vi "Configure.vi"(8 "error in (no error)":errorcluster, 10 "Msg in":T2, 11 "FakePressureController in":refnum<class "Tapedrive_ESP301.lvclass">) -> (0 "error out":errorcluster, 1 "new command":string, 2 "Msg out":T2, 3 "FakePressureController out":refnum<class "Tapedrive_ESP301.lvclass">)   [LabVIEW 2013, in "Tapedrive_ESP301.lvclass"]
uses:
  Tapedrive_ESP301.lvclass
  shared/OnOffTypeDef.ctl
  shared/CompressAndUpdate(Poly)/CompressAndUpdate(Numeric).vi
  shared/CompressAndUpdate(Poly)/CompressAndUpdate(Enum).vi
  shared/CompressAndUpdate(Poly)/CompressAndUpdate(String).vi
  BaseDriver/BaseDriver.lvclass
  BaseDriver/DriverMsg.ctl
panel:
  out "Error Code":i32[](array[numeric])
  out "Error Message":string
  out "velo":dbl(graph)
  out "Position (units)":dbl(graph)
  out "spreadsheet string":string
  out "found?":bool
  out "Settings.Velocity":T1
  out "Channel":string
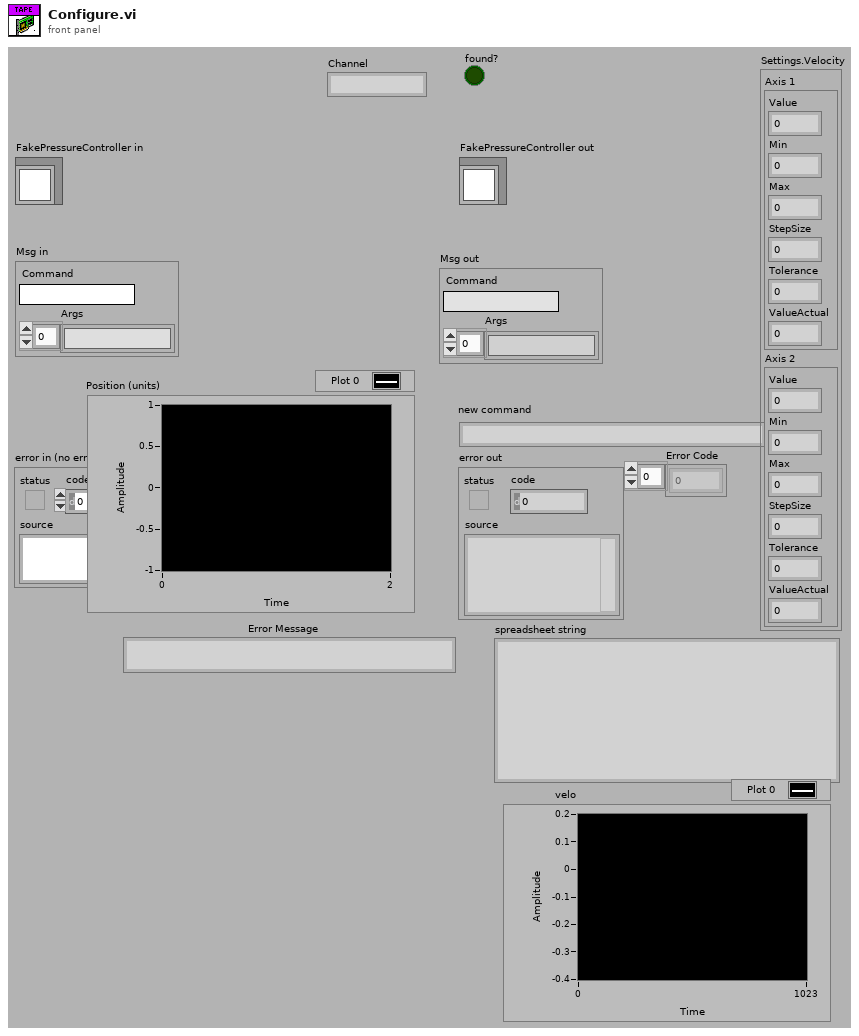
[diagram p1: front panel]
types:
  T1 = cluster{"Axis 1":cluster{"Value":dbl, "Min":dbl, "Max":dbl, "StepSize":dbl, "Tolerance":dbl, "ValueActual":dbl}, "Axis 2":cluster{"Value":dbl, "Min":dbl, "Max":dbl, "StepSize":dbl, "Tolerance":dbl, "ValueActual":dbl}}
  T2 = typedef "DriverMsg.ctl" = cluster{"Command":string, "Args":string[]}
  T3 = typedef "OnOffTypeDef.ctl" = enum16{"off", "on"}
  T4 = enum16{"Not referenced", "Homing", "Moving", "Ready"}
  T5 = typedef "Direction.ctl" = enum16{"Forward", "Backward", "Undefined"}
  T6 = typedef "Tapedrive_ESP301.lvclass/settingsCluster_TapeDrive_TypDef.ctl" = cluster{"devport":string, "tapepos":cluster{"Value":dbl, "Min":dbl, "Max":dbl, "StepSize":dbl, "Tolerance":dbl, "ValueActual":dbl}, "status":enum16{"Not referenced", "Homing", "Moving", "Ready"}, "inmotion":T3, "forwardaxis":i16, "backwardaxis":i16, "encoderaxis":i16, "Velocity":cluster{"Axis 1":cluster{"Value":dbl, "Min":dbl, "Max":dbl, "StepSize":dbl, "Tolerance":dbl, "ValueActual":dbl}, "Axis 2":cluster{"Value":dbl, "Min":dbl, "Max":dbl, "StepSize":dbl, "Tolerance":dbl, "ValueActual":dbl}}, "Acceleration":cluster{"Axis 1":cluster{"Value":dbl, "Min":dbl, "Max":dbl, "StepSize":dbl, "Tolerance":dbl, "ValueActual":dbl}, "Axis 2":cluster{"Value":dbl, "Min":dbl, "Max":dbl, "StepSize":dbl, "Tolerance":dbl, "ValueActual":dbl}}, "Decceleration":cluster{"Axis 1":cluster{"Value":dbl, "Min":dbl, "Max":dbl, "StepSize":dbl, "Tolerance":dbl, "ValueActual":dbl}, "Axis 2":cluster{"Value":dbl, "Min":dbl, "Max":dbl, "StepSize":dbl, "Tolerance":dbl, "ValueActual":dbl}}, "MaxAcceleration":cluster{"Axis 1":cluster{"Value":dbl, "Min":dbl, "Max":dbl, "StepSize":dbl, "Tolerance":dbl, "ValueActual":dbl}, "Axis 2":cluster{"Value":dbl, "Min":dbl, "Max":dbl, "StepSize":dbl, "Tolerance":dbl, "ValueActual":dbl}}, "MaxVelocity":cluster{"Axis 1":cluster{"Value":dbl, "Min":dbl, "Max":dbl, "StepSize":dbl, "Tolerance":dbl, "ValueActual":dbl}, "Axis 2":cluster{"Value":dbl, "Min":dbl, "Max":dbl, "StepSize":dbl, "Tolerance":dbl, "ValueActual":dbl}}, "VelocityFFG":cluster{"Axis 1":cluster{"Value":dbl, "Min":dbl, "Max":dbl, "StepSize":dbl, "Tolerance":dbl, "ValueActual":dbl}, "Axis 2":cluster{"Value":dbl, "Min":dbl, "Max":dbl, "StepSize":dbl, "Tolerance":dbl, "ValueActual":dbl}}, "AccelerationFFG":cluster{"Axis 1":cluster{"Value":dbl, "Min":dbl, "Max":dbl, "StepSize":dbl, "Tolerance":dbl, "ValueActual":dbl}, "Axis 2":cluster{"Value":dbl, "Min":dbl, "Max":dbl, "StepSize":dbl, "Tolerance":dbl, "ValueActual":dbl}}, "DACoffset":cluster{"Axis 1":cluster{"Value":dbl, "Min":dbl, "Max":dbl, "StepSize":dbl, "Tolerance":dbl, "ValueActual":dbl}, "Axis 2":cluster{"Value":dbl, "Min":dbl, "Max":dbl, "StepSize":dbl, "Tolerance":dbl, "ValueActual":dbl}}, "Power":cluster{"Axis 1":T3, "Axis 2":T3}, "ReductionRatio":cluster{"Value":dbl, "Min":dbl, "Max":dbl, "StepSize":dbl, "Tolerance":dbl, "ValueActual":dbl}, "Direction":T5, "Tension":T3, "TensionVelocity":cluster{"Axis 1":cluster{"Value":dbl, "Min":dbl, "Max":dbl, "StepSize":dbl, "Tolerance":dbl, "ValueActual":dbl}, "Axis 2":cluster{"Value":dbl, "Min":dbl, "Max":dbl, "StepSize":dbl, "Tolerance":dbl, "ValueActual":dbl}}, "TensionAcceleration":cluster{"Axis 1":cluster{"Value":dbl, "Min":dbl, "Max":dbl, "StepSize":dbl, "Tolerance":dbl, "ValueActual":dbl}, "Axis 2":cluster{"Value":dbl, "Min":dbl, "Max":dbl, "StepSize":dbl, "Tolerance":dbl, "ValueActual":dbl}}, "TensionDecceleration":cluster{"Axis 1":cluster{"Value":dbl, "Min":dbl, "Max":dbl, "StepSize":dbl, "Tolerance":dbl, "ValueActual":dbl}, "Axis 2":cluster{"Value":dbl, "Min":dbl, "Max":dbl, "StepSize":dbl, "Tolerance":dbl, "ValueActual":dbl}}, "MoveVelocity":cluster{"Axis 1":cluster{"Value":dbl, "Min":dbl, "Max":dbl, "StepSize":dbl, "Tolerance":dbl, "ValueActual":dbl}, "Axis 2":cluster{"Value":dbl, "Min":dbl, "Max":dbl, "StepSize":dbl, "Tolerance":dbl, "ValueActual":dbl}}, "MoveAcceleration":cluster{"Axis 1":cluster{"Value":dbl, "Min":dbl, "Max":dbl, "StepSize":dbl, "Tolerance":dbl, "ValueActual":dbl}, "Axis 2":cluster{"Value":dbl, "Min":dbl, "Max":dbl, "StepSize":dbl, "Tolerance":dbl, "ValueActual":dbl}}, "MoveDecceleration":cluster{"Axis 1":cluster{"Value":dbl, "Min":dbl, "Max":dbl, "StepSize":dbl, "Tolerance":dbl, "ValueActual":dbl}, "Axis 2":cluster{"Value":dbl, "Min":dbl, "Max":dbl, "StepSize":dbl, "Tolerance":dbl, "ValueActual":dbl}}, "MaxStepsize":cluster{"Value":dbl, "Min":dbl, "Max":dbl, "StepSize":dbl, "Tolerance":dbl, "ValueActual":dbl}, "Stepsize":cluster{"Value":dbl, "Min":dbl, "Max":dbl, "StepSize":dbl, "Tolerance":dbl, "ValueActual":dbl}, "GoStep":T3, "StopWait":T3, "stepnum":cluster{"Value":dbl, "Min":dbl, "Max":dbl, "StepSize":dbl, "Tolerance":dbl, "ValueActual":dbl}, "MoveIfScan":T3, "HomeEncoder":T3, "Timeout":cluster{"Value":dbl, "Min":dbl, "Max":dbl, "StepSize":dbl, "Tolerance":dbl, "ValueActual":dbl}, "TapeRelax":cluster{"Value":dbl, "Min":dbl, "Max":dbl, "StepSize":dbl, "Tolerance":dbl, "ValueActual":dbl}}
  T7 = cluster{"Axis 1":cluster{"Value":dbl, "Min":dbl, "Max":dbl, "StepSize":dbl, "Tolerance":dbl, "ValueActual":dbl}, "Axis 2":cluster{"Value":dbl, "Min":dbl, "Max":dbl, "StepSize":dbl, "Tolerance":dbl, "ValueActual":dbl}}[]
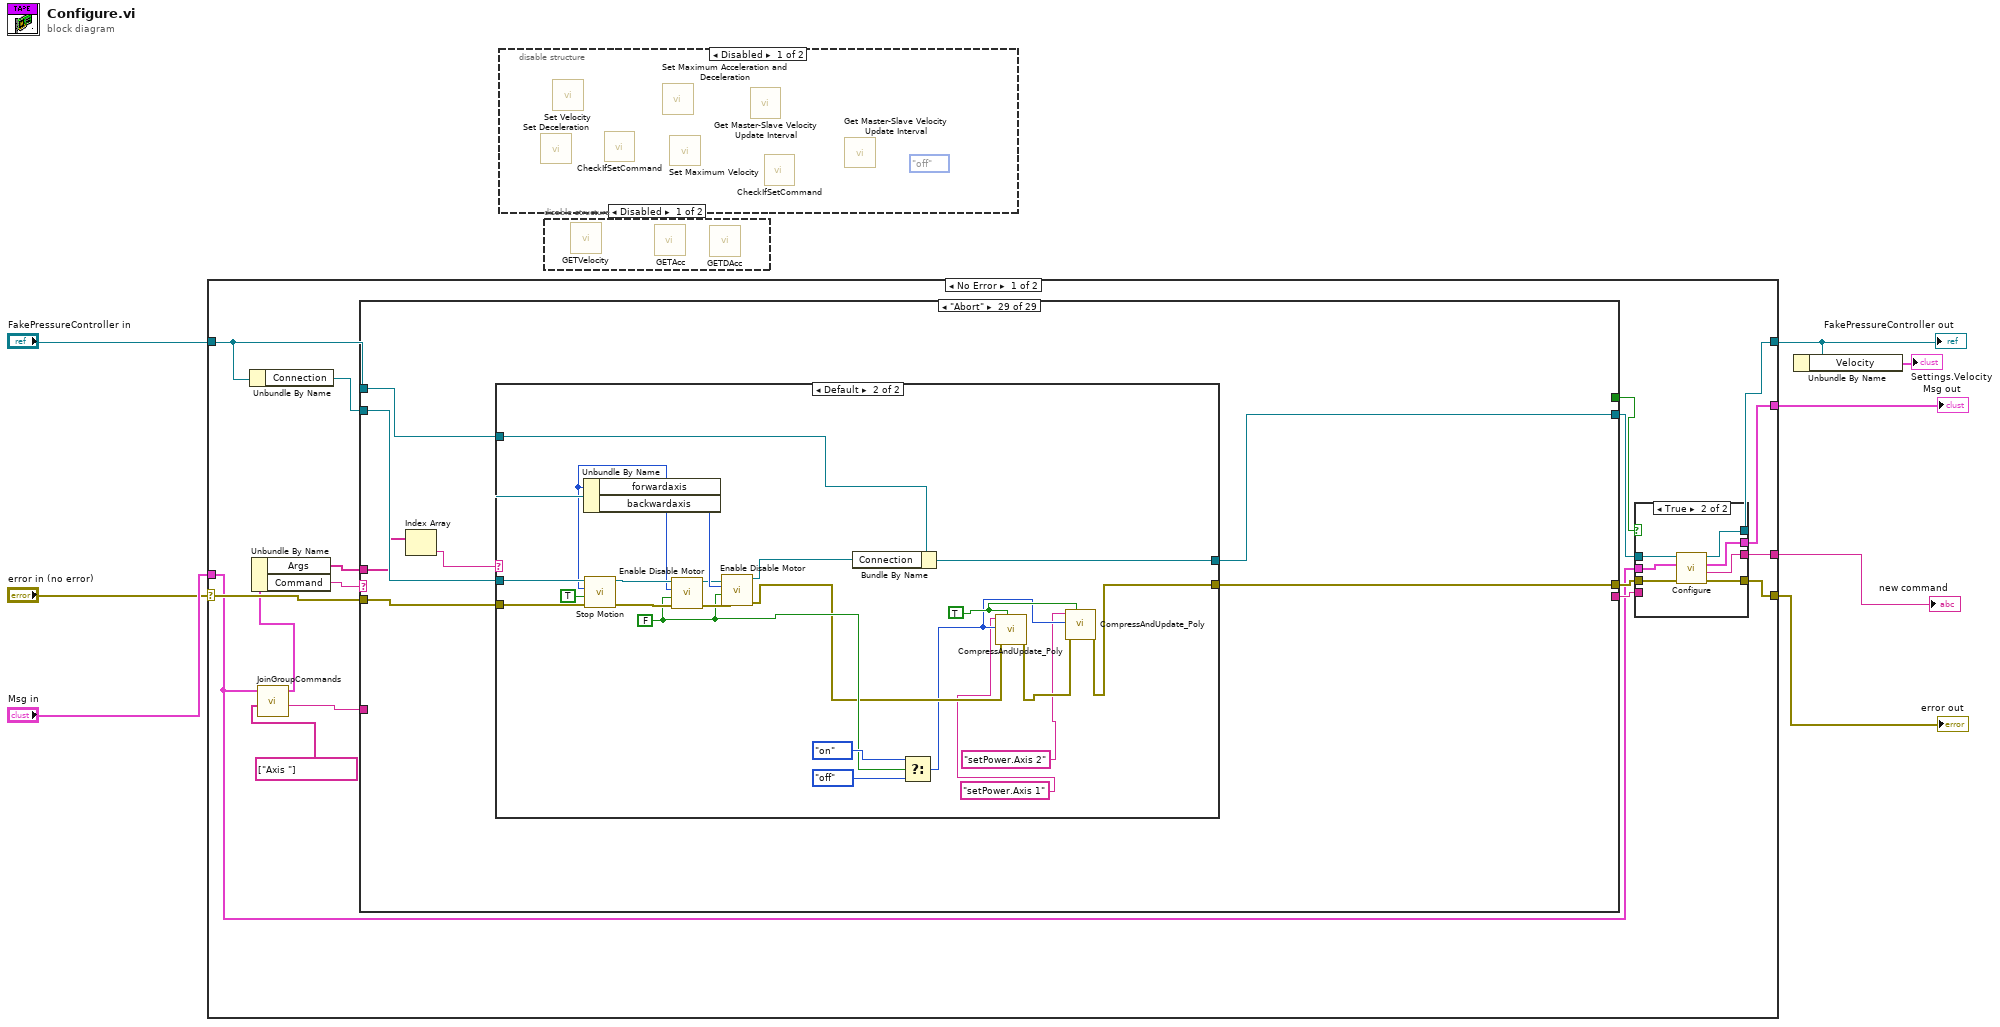
[diagram p0: block diagram]
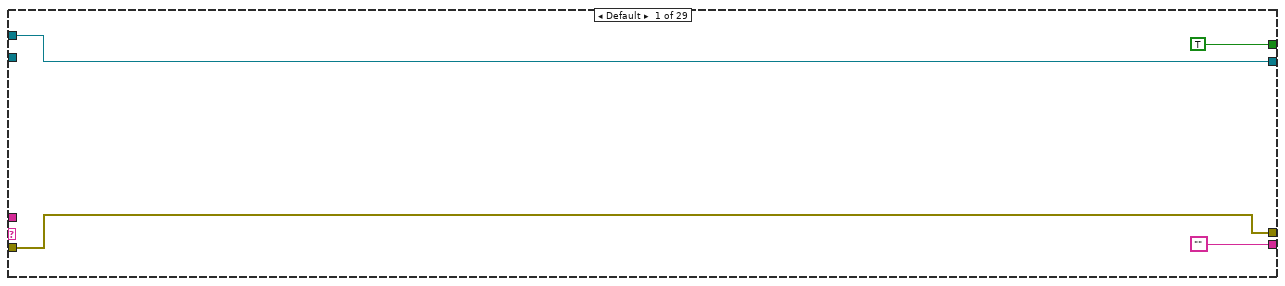
[diagram p5: hidden frame]
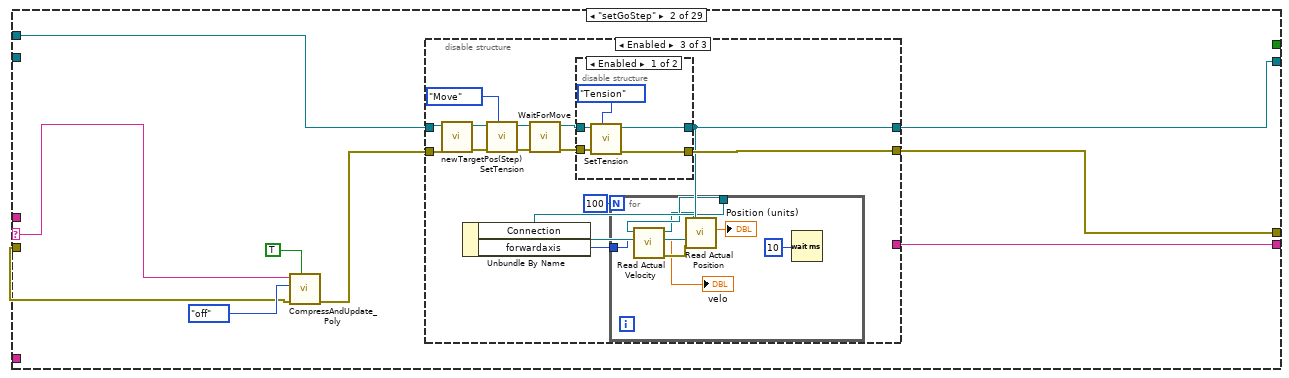
[diagram p6: hidden frame]
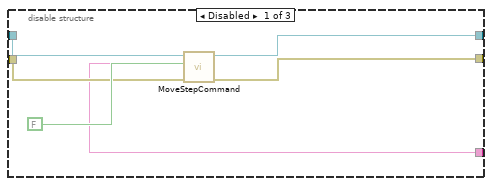
[diagram p7: hidden frame]
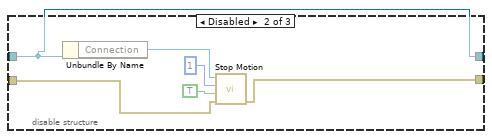
[diagram p8: hidden frame]
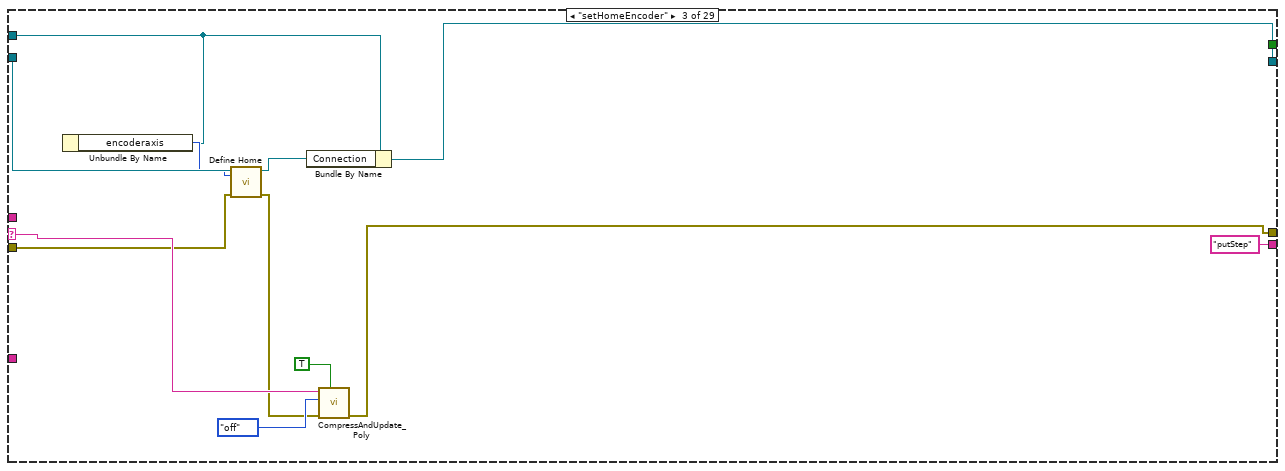
[diagram p10: hidden frame]
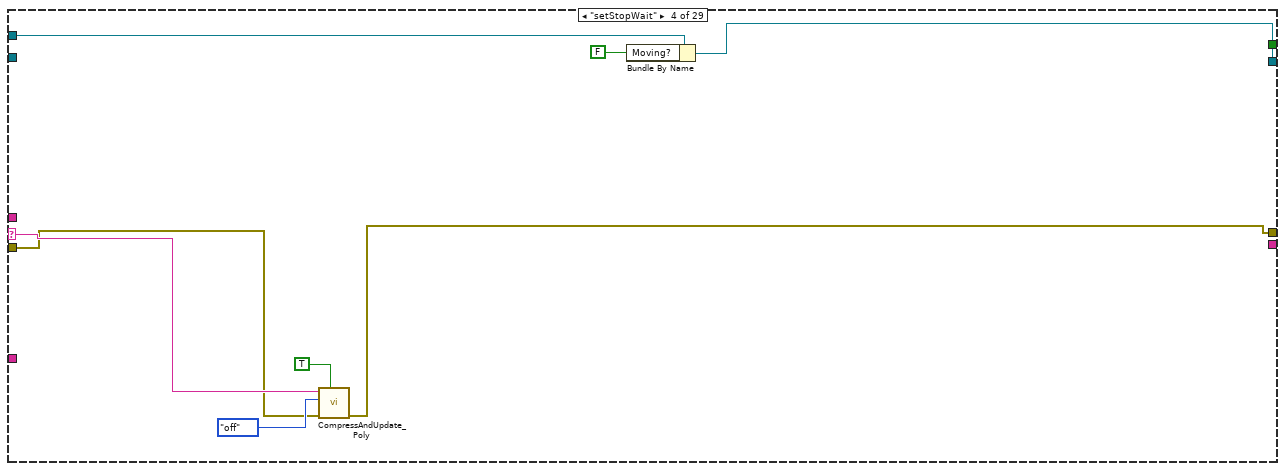
[diagram p11: hidden frame]
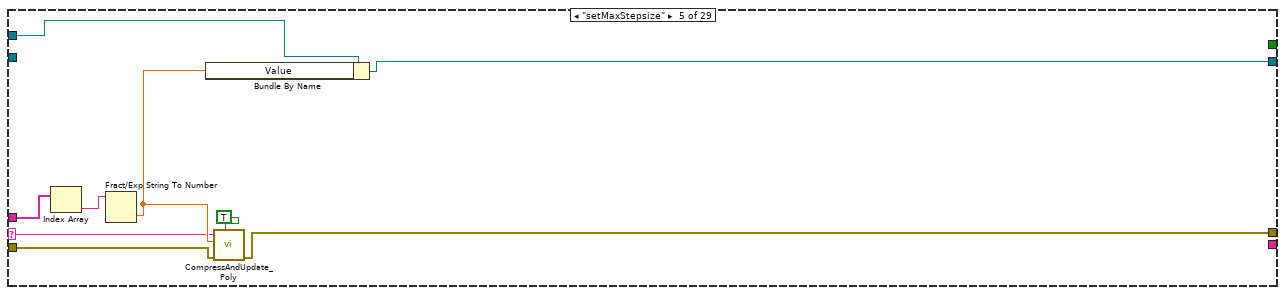
[diagram p12: hidden frame]
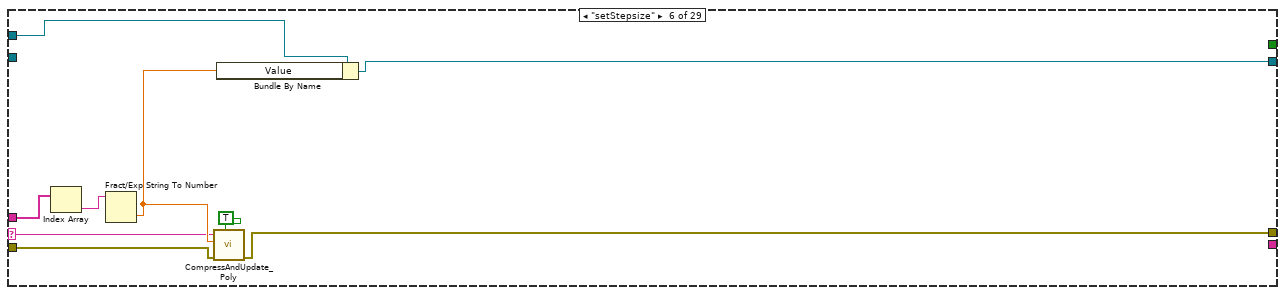
[diagram p13: hidden frame]
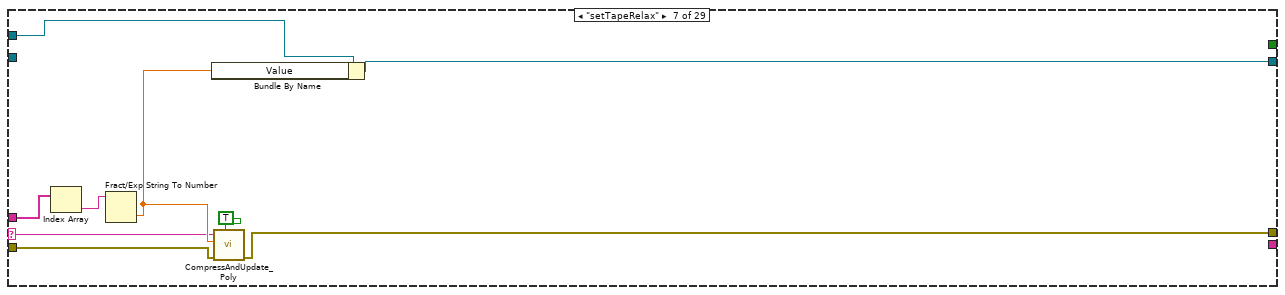
[diagram p14: hidden frame]
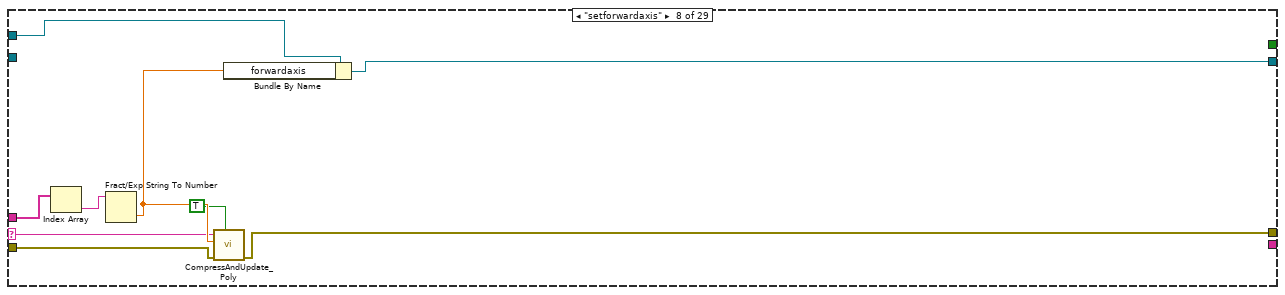
[diagram p15: hidden frame]
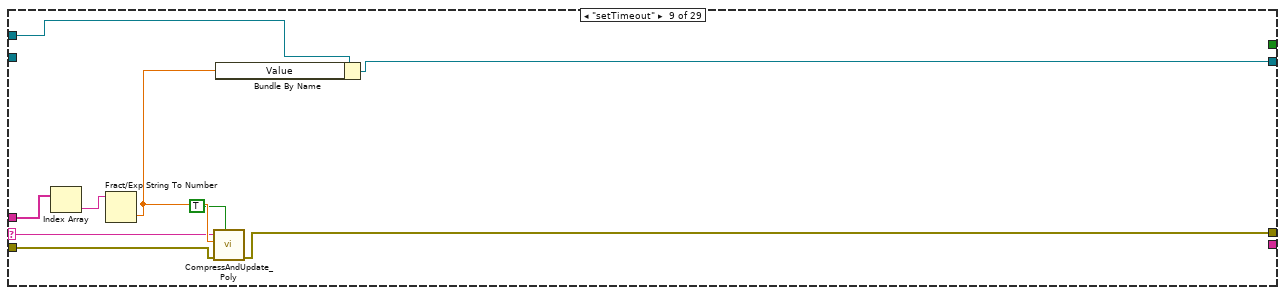
[diagram p16: hidden frame]
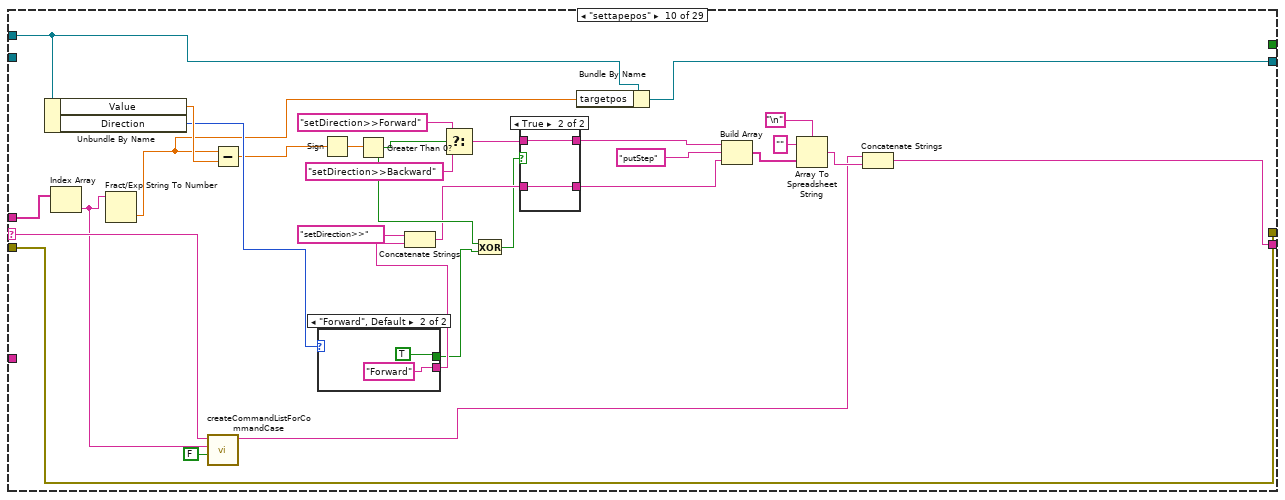
[diagram p17: hidden frame]
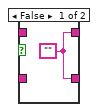
[diagram p18: hidden frame]
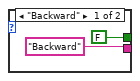
[diagram p19: hidden frame]
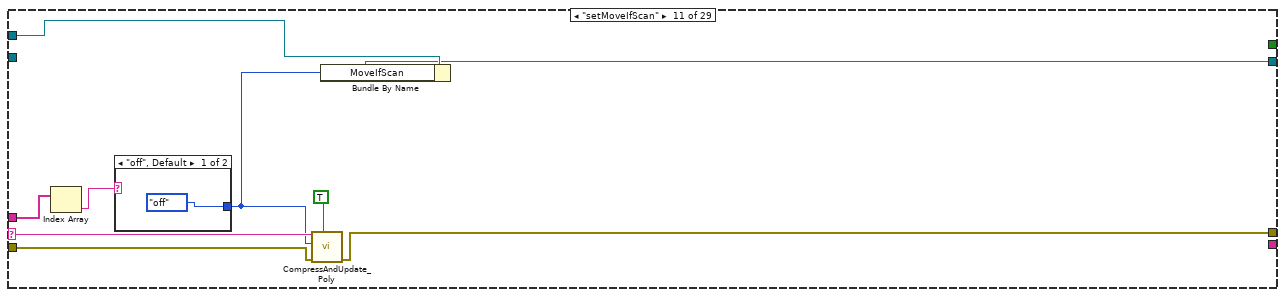
[diagram p20: hidden frame]
diagram:
  n1 = case shown="No Error" "error in (no error)" {
    selector: "error in (no error)" -> [w17 w958]
    tunnel: "FakePressureController in" -> [w14 w956]
    tunnel: [w24 w956] -> w2
    tunnel: [w22 w958] -> w5
    tunnel: "Msg in" -> [w9 w957]
    tunnel: [w20 w957] -> w4
    tunnel: [w18 _] -> w3
    frame No Error {
      n2 = Unbundle By Name(w14) -> ("Connection"=w13:refnum<visa-resource-name>)
      n3 = call "JoinGroupCommands.vi"("Seperator"=string[] ["Axis "], "Msg in"=w9) -> ("Seperator out"=w10:string, "Msg out"=w12:T2)  [unwired: 7 in, 1 out]
      n4 = Unbundle By Name(w12) -> ("Args"=w16:string[], "Command"=w15:string)
      n5 = case shown="\"Abort\"" w15 {
        selector: w15 -> [_ w42 w99 w108 w112 w121 w130 w139 w148 w172 w196 w205 w214 w224 w238 w270 w456 w480 w504 w687 w717 _ _ _ _ w803 _ _ _]
        tunnel: w17 -> [w39 w47 w93 w105 w111 w120 w129 w138 w147 w182 w195 w204 w213 w223 w229 w278 w465 w476 w506 w676 w701 w721 w727 w732 w742 w815 w830 w902 w928]
        tunnel: w16 -> [_ _ _ _ w115 w124 w133 w142 w151 w183 w197 w208 w217 w225 w240 w277 w464 w487 w515 w673 w708 w723 _ w731 _ w814 _ w905 w926]
        tunnel: w14 -> [w40 w45 w91 w103 w117 w126 w135 w144 w153 w177 w199 w210 w219 w227 w232 w260 w458 w483 w493 w680 w693 w720 w726 w733 w737 w811 w825 w897 w930]
        tunnel: [w40 w44 w90 w102 w116 w125 w134 w143 w152 w176 w198 w209 w218 w226 w241 w271 w457 w481 w508 w678 w709 w719 w725 w733 w734 w810 w822 w888 w931] -> w25
        tunnel: ["" ("Complete") w41 "putStep" ("spreadsheet string") _ _ _ _ _ _ w167 _ _ _ _ w235 w264 w440 w477 w509 w681 w711 _ _ _ w743 _ w831 w900 _] -> w19
        tunnel: [w39 w46 w96 w104 w110 w119 w128 w137 w146 w182 w194 w203 w212 w222 w234 w259 w443 w475 w491 w662 w698 w718 w724 w732 w736 w804 w824 w889 w927] -> w23
        tunnel: [TRUE _ _ _ _ _ _ _ _ _ _ _ _ _ _ _ _ _ _ _ _ _ _ _ _ _ _ _ _] -> w21
        tunnel: w13 -> [_ _ w95 _ _ _ _ _ _ _ _ _ _ _ w231 w279 w466 _ w505 w677 w702 _ _ _ w740 w819 w828 w904 w929]
        tunnel: w10 -> [_ _ _ _ _ _ _ _ _ _ _ _ _ _ _ w275 w462 _ w513 w685 w715 _ _ _ _ _ _ _ _]
        frame Default {
        }
        frame "setGoStep" {
          n6 = call-poly "CompressAndUpdate_Poly.vi"("force CVT update (false)"=TRUE, "error in"=w47, "enum variant"=OnOffTypeDef."off" ("inmotion"), "command or variable name"=w42) -> ("error out"=w43:errorcluster)  [unwired: 7 in]
          n7 = disable-structure shown="Enabled" {
            disable-tunnel: [w55 w56 w72] -> w46
            disable-tunnel: w45 -> [w54 w59 w67]
            disable-tunnel: [w53 w59 w64] -> w44
            disable-tunnel: w43 -> [w51 w57 w74]
            disable-tunnel: [w50 _ _] -> w41
            frame Disabled {
              n8 = call "MoveStepCommand.vi"("error in (no error)"=w51, "MultiCVT"=FALSE, "Tapedrive_ESP301 in"=w54) -> ("error out"=w55:errorcluster, "String"=w50:string, "Tapedrive_ESP301.lvclass"=w53:refnum<class "Tapedrive_ESP301.lvclass">)  [unwired: 6 in]
            }
            frame Disabled {
              n9 = Unbundle By Name(w59) -> ("Connection"=w58:refnum<visa-resource-name>)
              n10 = call <instrlib>:"Stop Motion.vi"("error in (no error)"=w57, "Stop all axes (F)"=TRUE, "Axis (1)"=1, "VISA resource name"=w58) -> ("error out"=w56:errorcluster)  [unwired: 2 in, 1 out]
            }
            frame Enabled {
              n11 = call "newTargetPos(Step).vi"("Tapedrive_ESP301 in"=w67) -> ("Tapedrive_ESP301 out"=w66:refnum<class "Tapedrive_ESP301.lvclass">)  [unwired: 9 in, 1 out]
              n12 = call "SetTension.vi"("command"=enum16{"Move", "Tension"}."Move", "error in (no error)"=w74, "Tapedrive_ESP301 in"=w66) -> ("error out"=w69:errorcluster, "Tapedrive_ESP301 out"=w71:refnum<class "Tapedrive_ESP301.lvclass">)  [unwired: 7 in]
              n13 = call-dynamic "WaitForMove.vi"("error in (no error)"=w69, "Tapedrive Object"=w71) -> ("error out (no error)"=w68:errorcluster, "Tapedrive Object 2"=w70:refnum<class "Tapedrive_ESP301.lvclass">)  [unwired: 7 in, 1 out]
              n14 = disable-structure shown="Enabled" {
                disable-tunnel: [w86 w88] -> w64
                disable-tunnel: [w84 w87] -> w72
                disable-tunnel: w70 -> [w83 w88]
                disable-tunnel: w68 -> [w82 w87]
                frame Enabled {
                  n15 = call "SetTension.vi"("command"=enum16{"Move", "Tension"}."Tension", "error in (no error)"=w82, "Tapedrive_ESP301 in"=w83) -> ("error out"=w84:errorcluster, "Tapedrive_ESP301 out"=w86:refnum<class "Tapedrive_ESP301.lvclass">)  [unwired: 7 in]
                }
                frame Disabled {
                }
              }
              n16 = Unbundle By Name(w64) -> ("Connection"=w63:refnum<visa-resource-name>, "forwardaxis"=w62:i16)
              n17 = for {
                N: 100 -> [_]
                tunnel: w63 -> [w78]
                tunnel: w62 -> [w76]
                n18 = call <instrlib>:"Read Actual Velocity.vi"("Axis (1)"=w76, "VISA resource name"=w78) -> ("error out"=w79:errorcluster, "Velocity (units/s)"=→"velo":dbl, "VISA resource name out"=w77:refnum<visa-resource-name>)  [unwired: 3 in]
                n19 = call <instrlib>:"Read Actual Position.vi"("error in (no error)"=w79, "VISA resource name"=w77) -> ("Position (units)"=→"Position (units)":dbl)  [unwired: 3 in, 2 out]
                n20 = Wait (ms)(milliseconds to wait=u32 10) -> ()  [unwired: 1 out]
              }
            }
          }
        }
        frame "setHomeEncoder" {
          n21 = Unbundle By Name(w91) -> ("encoderaxis"=w94:i16)
          n22 = call <instrlib>:"Define Home.vi"("error in (no error)"=w93, "Axis (1)"=w94, "VISA resource name"=w95) -> ("error out"=w92:errorcluster, "VISA resource name out"=w89:refnum<visa-resource-name>)  [unwired: 3 in]
          n23 = Bundle By Name(cluster=w91, "Connection"=w89) -> (w90:refnum<class "Tapedrive_ESP301.lvclass">)
          n24 = call-poly "CompressAndUpdate_Poly.vi"("force CVT update (false)"=TRUE, "error in"=w92, "enum variant"=OnOffTypeDef."off" ("inmotion"), "command or variable name"=w99) -> ("error out"=w96:errorcluster)  [unwired: 7 in]
        }
        frame "setStopWait" {
          n25 = call-poly "CompressAndUpdate_Poly.vi"("force CVT update (false)"=TRUE, "error in"=w105, "enum variant"=OnOffTypeDef."off" ("inmotion"), "command or variable name"=w108) -> ("error out"=w104:errorcluster)  [unwired: 7 in]
          n26 = Bundle By Name(cluster=w103, "Moving?"=FALSE ("Wait for Step")) -> (w102:refnum<class "Tapedrive_ESP301.lvclass">)
        }
        frame "setMaxStepsize" {
          n27 = Index Array(array=w115) -> (element=w114:string)  [unwired: 1 in]
          n28 = Fract/Exp String To Number(string=w114) -> (number=w113:dbl)  [unwired: 3 in, 1 out]
          n29 = Bundle By Name(cluster=w117, "Value"=w113) -> (w116:refnum<class "Tapedrive_ESP301.lvclass">)
          n30 = call-poly "CompressAndUpdate_Poly.vi"("force CVT update (false)"=TRUE, "error in"=w111, "Numeric"=w113, "command or variable name"=w112) -> ("error out"=w110:errorcluster)  [unwired: 7 in]
        }
        frame "setStepsize" {
          n31 = Index Array(array=w124) -> (element=w123:string)  [unwired: 1 in]
          n32 = Fract/Exp String To Number(string=w123) -> (number=w122:dbl)  [unwired: 3 in, 1 out]
          n33 = call-poly "CompressAndUpdate_Poly.vi"("force CVT update (false)"=TRUE, "error in"=w120, "Numeric"=w122, "command or variable name"=w121) -> ("error out"=w119:errorcluster)  [unwired: 7 in]
          n34 = Bundle By Name(cluster=w126, "Value"=w122) -> (w125:refnum<class "Tapedrive_ESP301.lvclass">)
        }
        frame "setTapeRelax" {
          n35 = Index Array(array=w133) -> (element=w132:string)  [unwired: 1 in]
          n36 = Fract/Exp String To Number(string=w132) -> (number=w131:dbl)  [unwired: 3 in, 1 out]
          n37 = Bundle By Name(cluster=w135, "Value"=w131) -> (w134:refnum<class "Tapedrive_ESP301.lvclass">)
          n38 = call-poly "CompressAndUpdate_Poly.vi"("force CVT update (false)"=TRUE, "error in"=w129, "Numeric"=w131, "command or variable name"=w130) -> ("error out"=w128:errorcluster)  [unwired: 7 in]
        }
        frame "setforwardaxis" {
          n39 = Index Array(array=w142) -> (element=w141:string)  [unwired: 1 in]
          n40 = Fract/Exp String To Number(string=w141) -> (number=w140:dbl)  [unwired: 3 in, 1 out]
          n41 = call-poly "CompressAndUpdate_Poly.vi"("force CVT update (false)"=TRUE, "error in"=w138, "Numeric"=w140, "command or variable name"=w139) -> ("error out"=w137:errorcluster)  [unwired: 7 in]
          n42 = Bundle By Name(cluster=w144, "forwardaxis"=w140) -> (w143:refnum<class "Tapedrive_ESP301.lvclass">)
        }
        frame "setTimeout" {
          n43 = Index Array(array=w151) -> (element=w150:string)  [unwired: 1 in]
          n44 = Fract/Exp String To Number(string=w150) -> (number=w149:dbl)  [unwired: 3 in, 1 out]
          n45 = call-poly "CompressAndUpdate_Poly.vi"("force CVT update (false)"=TRUE, "error in"=w147, "Numeric"=w149, "command or variable name"=w148) -> ("error out"=w146:errorcluster)  [unwired: 7 in]
          n46 = Bundle By Name(cluster=w153, "Value"=w149) -> (w152:refnum<class "Tapedrive_ESP301.lvclass">)
        }
        frame "settapepos" {
          n47 = Unbundle By Name(w177) -> ("Value"=w181:dbl, "Direction"=w164:T5)
          n48 = Index Array(array=w183) -> (element=w171:string)  [unwired: 1 in]
          n49 = Fract/Exp String To Number(string=w171) -> (number=w155:dbl)  [unwired: 3 in, 1 out]
          n50 = call "createCommandListForCommandCase.vi"("immediate Check (only once)"=FALSE, "setvalue"=w171, "command"=w172) -> ("new commands"=w168:string)  [unwired: 8 in]
          n51 = Subtract(x=w155, y=w181) -> (x-y=w154:dbl)
          n52 = case shown="\"Forward\", Default" w164 {
            tunnel: ["Backward" "Forward"] -> w163
            tunnel: [FALSE TRUE] -> w161
            frame "Backward" {
            }
            frame "Forward", Default {
            }
          }
          n53 = Sign(1:w154) -> (0:w180:dbl)
          n54 = Greater Than 0?(x=w180) -> (x > 0?=w162:bool)
          n55 = Concatenate Strings("setDirection>>", w163) -> (w158:string)
          n56 = Select(t="setDirection>>Forward", s=w162, f="setDirection>>Backward") -> (s? t:f=w160:string)
          n57 = Exclusive Or(1:w161, 2:w162) -> (0:w156:bool)
          n58 = case shown="True" w156 {
            tunnel: w160 -> [_ w186]
            tunnel: [w184 w186] -> w159
            tunnel: w158 -> [_ w185]
            tunnel: [w184 w185] -> w157
            frame False {
              w184 = ""
            }
            frame True {
            }
          }
          n59 = Bundle By Name(cluster=w177, "targetpos"=w155) -> (w176:refnum<class "Tapedrive_ESP301.lvclass">)
          n60 = Build Array(w159, "putStep", w157) -> (w175:string[])
          n61 = Array To Spreadsheet String(delimiter (Tab)="\n", array=w175, 3:"" ("format string")) -> (spreadsheet string=w169:string)
          n62 = Concatenate Strings(w168, w169) -> (w167:string)
        }
        frame "setMoveIfScan" {
          n63 = Index Array(array=w197) -> (element=w192:string)  [unwired: 1 in]
          n64 = case shown="\"off\", Default" w192 {
            tunnel: [OnOffTypeDef."off" ("inmotion") OnOffTypeDef."on" ("inmotion")] -> w191
            frame "off", Default {
            }
            frame "on" {
            }
          }
          n65 = call-poly "CompressAndUpdate_Poly.vi"("force CVT update (false)"=TRUE, "error in"=w195, "enum variant"=w191, "command or variable name"=w196) -> ("error out"=w194:errorcluster)  [unwired: 7 in]
          n66 = Bundle By Name(cluster=w199, "MoveIfScan"=w191) -> (w198:refnum<class "Tapedrive_ESP301.lvclass">)
        }
        frame "setbackwardaxis" {
          n67 = Index Array(array=w208) -> (element=w207:string)  [unwired: 1 in]
          n68 = Fract/Exp String To Number(string=w207) -> (number=w206:dbl)  [unwired: 3 in, 1 out]
          n69 = call-poly "CompressAndUpdate_Poly.vi"("force CVT update (false)"=TRUE, "error in"=w204, "Numeric"=w206, "command or variable name"=w205) -> ("error out"=w203:errorcluster)  [unwired: 7 in]
          n70 = Bundle By Name(cluster=w210, "backwardaxis"=w206) -> (w209:refnum<class "Tapedrive_ESP301.lvclass">)
        }
        frame "setencoderaxis" {
          n71 = Index Array(array=w217) -> (element=w216:string)  [unwired: 1 in]
          n72 = Fract/Exp String To Number(string=w216) -> (number=w215:dbl)  [unwired: 3 in, 1 out]
          n73 = call-poly "CompressAndUpdate_Poly.vi"("force CVT update (false)"=TRUE, "error in"=w213, "Numeric"=w215, "command or variable name"=w214) -> ("error out"=w212:errorcluster)  [unwired: 7 in]
          n74 = Bundle By Name(cluster=w219, "encoderaxis"=w215) -> (w218:refnum<class "Tapedrive_ESP301.lvclass">)
        }
        frame "setdevport" {
          n75 = Index Array(array=w225) -> (element=w221:string)  [unwired: 1 in]
          n76 = call-poly "CompressAndUpdate_Poly.vi"("force CVT update (false)"=TRUE, "error in"=w223, "String"=w221, "command or variable name"=w224) -> ("error out"=w222:errorcluster)  [unwired: 7 in]
          n77 = Bundle By Name(cluster=w227, "devport"=w221) -> (w226:refnum<class "Tapedrive_ESP301.lvclass">)
        }
        frame "setTension" {
          # "TODO: tension off??"
          n78 = Index Array(array=w240) -> (element=w237:string)  [unwired: 1 in]
          n79 = Unbundle By Name(w232) -> ("forwardaxis"=w230:i16)
          n80 = call "createCommandListForCommandCase.vi"("setvalue"=w237, "command"=w238) -> ("new commands"=w236:string)  [unwired: 9 in]
          n81 = case shown="\"on\"" w237 {
            tunnel: w236 -> [w247 w253]
            tunnel: [w247 w251] -> w235
            tunnel: [OnOffTypeDef."off" ("Tension") OnOffTypeDef."on" ("Tension")] -> w233
            tunnel: w231 -> [w245 _]
            tunnel: w230 -> [w244 _]
            tunnel: w229 -> [w243 w249]
            tunnel: [w242 w249] -> w228
            frame "off", Default {
              n82 = call <instrlib>:"Stop Motion.vi"("error in (no error)"=w243, "Stop all axes (F)"=TRUE, "Axis (1)"=w244, "VISA resource name"=w245) -> ("error out"=w242:errorcluster)  [unwired: 2 in, 1 out]
            }
            frame "on" {
              n83 = Concatenate Strings(w253, "putTension" ("string")) -> (w251:string)
            }
          }
          n84 = call-poly "CompressAndUpdate_Poly.vi"("force CVT update (false)"=TRUE, "error in"=w228, "enum variant"=w233, "command or variable name"=w238) -> ("error out"=w234:errorcluster)  [unwired: 7 in]
          n85 = Bundle By Name(cluster=w232, "Tension"=w233) -> (w241:refnum<class "Tapedrive_ESP301.lvclass">)
        }
        frame "setAcceleration", "setAccelerationFFG", "setDecceleration", "setMaxAcceleration", "setMaxVelocity", "setVelocity", "setVelocityFFG" {
          n86 = call "reBuildJoindCommand.vi"("number of group elements (0)"=1, "Args"=w277, "Command 2"=w270) -> ("Arg"=w273:string, "Command"=w269:string)
          n87 = call "CheckIfSetCommand.vi"("Command"=w270) -> ("variable"=w261:string)  [unwired: 2 out]
          n88 = call "getSeperator.vi"("Channel Seperator (\"\")"=w275, "Command"=w269) -> ("Channel"=w254:string, "Seperator (e.g. \"Channel1\")"=w258:string)  [unwired: 8 in]
          "Channel" <- w258
          n89 = call "AxisNameTonumber.vi"("Channel"=w254, "Tapedrive_ESP301 in"=w260) -> ("Axis No."=w256:i16, "Tapedrive_ESP301 out"=w255:refnum<class "Tapedrive_ESP301.lvclass">)  [unwired: 8 in]
          n90 = Fract/Exp String To Number(string=w273) -> (number=w274:dbl)  [unwired: 3 in, 1 out]
          n91 = case shown="\"VelocityFFG\"" w261 {
            tunnel: w279 -> [w300 w321 w342 w363 w384 w405 w426]
            tunnel: w278 -> [w299 w320 w340 w361 w379 w403 w423]
            tunnel: w256 -> [w294 w317 w337 w357 w382 w400 w420]
            tunnel: w274 -> [w298 w316 w341 w362 w378 w404 w422]
            tunnel: [w282 w303 w325 w345 w366 w387 w408] -> w267
            tunnel: [w290 w306 w328 w351 w368 w389 w411] -> w268
            tunnel: [w295 w315 w338 w358 w381 w401 w424] -> w263
            tunnel: 100 -> [w280 w301 w322 w343 w364 w385 w406]
            tunnel: w255 -> [w292 w310 w330 w349 w371 w394 w413]
            tunnel: w258 -> [w293 w305 w327 w347 w369 w390 w410]
            tunnel: [w291 w309 w329 w348 w370 w393 w412] -> w262
            tunnel: [w281 w302 w324 w344 w365 w386 w407] -> w257
            frame "Velocity", Default {
              n92 = call <instrlib>:"Set Velocity.vi"("error in (no error)"=w299, "Velocity (units/s)"=w298, "Axis (1)"=w294, "VISA resource name"=w300) -> ("error out"=w296:errorcluster, "VISA resource name out"=w297:refnum<visa-resource-name>)  [unwired: 2 in]
              n93 = Unbundle By Name(w292) -> ("Velocity"=w285:T1)
              n94 = call "Get Velocity_CK.vi"("error in (no error)"=w296, "Wait before read (0ms)"=w280, "Axis (1)"=w294, "VISA resource name"=w297) -> ("error out"=w283:errorcluster, "Velocity (units/s)"=w290:dbl, "VISA resource name out"=w295:refnum<visa-resource-name>)  [unwired: 1 in]
              n95 = Concatenate Strings(w293, ".Value" ("string")) -> (w288:string)
              n96 = call "Set Cluster Element by Name__ogtk_TS.vi"("error in (no error)"=w283, "Element Name (\"\": New Element Data Name)"=w288, "New Element Value"=w290, "Cluster"=w285) -> ("error out"=w287:errorcluster, "found?"=w281:bool, "VCluster out"=w286:variant)  [unwired: 5 in]
              n97 = Variant To Data(error in=w287, type=w285, Variant=w286) -> (data=w284:T1, error out=w282:errorcluster)
              n98 = Bundle By Name(cluster=w292, "Velocity"=w284) -> (w291:refnum<class "Tapedrive_ESP301.lvclass">)
            }
            frame "Acceleration" {
              n99 = call <instrlib>:"Set Acceleration.vi"("error in (no error)"=w320, "Acceleration (0 units/s²)"=w316, "Axis (1)"=w317, "VISA resource name"=w321) -> ("error out"=w319:errorcluster, "VISA resource name out"=w318:refnum<visa-resource-name>)  [unwired: 2 in]
              n100 = Unbundle By Name(w310) -> ("Acceleration"=w308:T1)
              n101 = call "Get Acceleration_CK.vi"("error in (no error)"=w319, "Wait before read (0ms)"=w301, "Axis (1)"=w317, "VISA resource name"=w318) -> ("error out"=w304:errorcluster, "Acceleration (units/s²)"=w306:dbl, "VISA resource name out"=w315:refnum<visa-resource-name>)  [unwired: 1 in]
              n102 = Concatenate Strings(w305, ".Value" ("string")) -> (w313:string)
              n103 = call "Set Cluster Element by Name__ogtk_TS.vi"("error in (no error)"=w304, "Element Name (\"\": New Element Data Name)"=w313, "New Element Value"=w306, "Cluster"=w308) -> ("error out"=w312:errorcluster, "found?"=w302:bool, "VCluster out"=w311:variant)  [unwired: 5 in]
              n104 = Variant To Data(error in=w312, type=w308, Variant=w311) -> (data=w307:T1, error out=w303:errorcluster)
              n105 = Bundle By Name(cluster=w310, "Acceleration"=w307) -> (w309:refnum<class "Tapedrive_ESP301.lvclass">)
            }
            frame "Decceleration" {
              n106 = call <instrlib>:"Set Deceleration.vi"("error in (no error)"=w340, "Deceleration (0 units/s²)"=w341, "Axis (1)"=w337, "VISA resource name"=w342) -> ("error out"=w323:errorcluster, "VISA resource name out"=w339:refnum<visa-resource-name>)  [unwired: 2 in]
              n107 = Unbundle By Name(w330) -> ("Decceleration"=w336:T1)
              n108 = call "Get Deceleration_CK.vi"("error in (no error)"=w323, "Wait before read (0ms)"=w322, "Axis (1)"=w337, "VISA resource name"=w339) -> ("error out"=w326:errorcluster, "Deceleration (units/s²)"=w328:dbl, "VISA resource name out"=w338:refnum<visa-resource-name>)  [unwired: 1 in]
              n109 = Concatenate Strings(w327, ".Value" ("string")) -> (w334:string)
              n110 = call "Set Cluster Element by Name__ogtk_TS.vi"("error in (no error)"=w326, "Element Name (\"\": New Element Data Name)"=w334, "New Element Value"=w328, "Cluster"=w336) -> ("error out"=w333:errorcluster, "found?"=w324:bool, "VCluster out"=w332:variant)  [unwired: 5 in]
              n111 = Variant To Data(error in=w333, type=w336, Variant=w332) -> (data=w331:T1, error out=w325:errorcluster)
              n112 = Bundle By Name(cluster=w330, "Decceleration"=w331) -> (w329:refnum<class "Tapedrive_ESP301.lvclass">)
            }
            frame "MaxVelocity" {
              n113 = call <instrlib>:"Set Maximum Velocity.vi"("error in (no error)"=w361, "Maximum Velocity (0 units/s)"=w362, "Axis (1)"=w357, "VISA resource name"=w363) -> ("error out"=w360:errorcluster, "VISA resource name out"=w359:refnum<visa-resource-name>)  [unwired: 2 in]
              n114 = Unbundle By Name(w349) -> ("MaxVelocity"=w350:T1)
              n115 = call "Get Maximum Velocity_CK.vi"("error in (no error)"=w360, "Wait before read (0ms)"=w343, "Axis (1)"=w357, "VISA resource name"=w359) -> ("error out"=w346:errorcluster, "Maximum Velocity (units/s)"=w351:dbl, "VISA resource name out"=w358:refnum<visa-resource-name>)  [unwired: 1 in]
              n116 = Concatenate Strings(w347, ".Value" ("string")) -> (w355:string)
              n117 = call "Set Cluster Element by Name__ogtk_TS.vi"("error in (no error)"=w346, "Element Name (\"\": New Element Data Name)"=w355, "New Element Value"=w351, "Cluster"=w350) -> ("error out"=w354:errorcluster, "found?"=w344:bool, "VCluster out"=w353:variant)  [unwired: 5 in]
              n118 = Variant To Data(error in=w354, type=w350, Variant=w353) -> (data=w352:T1, error out=w345:errorcluster)
              n119 = Bundle By Name(cluster=w349, "MaxVelocity"=w352) -> (w348:refnum<class "Tapedrive_ESP301.lvclass">)
            }
            frame "MaxAcceleration" {
              n120 = call <instrlib>:"Set Maximum Acceleration and Deceleration.vi"("error in (no error)"=w379, "Acceleration (0 units/s²)"=w378, "Axis (1)"=w382, "VISA resource name"=w384) -> ("error out"=w380:errorcluster, "VISA resource name out"=w383:refnum<visa-resource-name>)  [unwired: 2 in]
              n121 = Unbundle By Name(w371) -> ("MaxAcceleration"=w377:T1)
              n122 = call "Get Maximum Acceleration and Deceleration_CK.vi"("error in (no error)"=w380, "Wait before read (0ms)"=w364, "Axis (1)"=w382, "VISA resource name"=w383) -> ("error out"=w367:errorcluster, "Acceleration (units/s²)"=w368:dbl, "VISA resource name out"=w381:refnum<visa-resource-name>)  [unwired: 1 in]
              n123 = Concatenate Strings(w369, ".Value" ("string")) -> (w375:string)
              n124 = call "Set Cluster Element by Name__ogtk_TS.vi"("error in (no error)"=w367, "Element Name (\"\": New Element Data Name)"=w375, "New Element Value"=w368, "Cluster"=w377) -> ("error out"=w374:errorcluster, "found?"=w365:bool, "VCluster out"=w373:variant)  [unwired: 5 in]
              n125 = Variant To Data(error in=w374, type=w377, Variant=w373) -> (data=w372:T1, error out=w366:errorcluster)
              n126 = Bundle By Name(cluster=w371, "MaxAcceleration"=w372) -> (w370:refnum<class "Tapedrive_ESP301.lvclass">)
            }
            frame "VelocityFFG" {
              n127 = Unbundle By Name(w394) -> ("VelocityFFG"=w391:T1)
              n128 = call <instrlib>:"Set Velocity Feed-Forward Gain.vi"("error in (no error)"=w403, "Velocity feed-forward gain factor (0)"=w404, "Axis (1)"=w400, "VISA resource name"=w405) -> ("error out"=w399:errorcluster, "VISA resource name out"=w402:refnum<visa-resource-name>)  [unwired: 2 in]
              n129 = call "Get Velocity Feed-Forward Gain_CK.vi"("error in (no error)"=w399, "Wait before read (0ms)"=w385, "Axis (1)"=w400, "VISA resource name"=w402) -> ("error out"=w388:errorcluster, "Gain"=w389:dbl, "VISA resource name out"=w401:refnum<visa-resource-name>)  [unwired: 1 in]
              n130 = Concatenate Strings(w390, ".Value" ("string")) -> (w397:string)
              n131 = call "Set Cluster Element by Name__ogtk_TS.vi"("error in (no error)"=w388, "Element Name (\"\": New Element Data Name)"=w397, "New Element Value"=w389, "Cluster"=w391) -> ("error out"=w396:errorcluster, "found?"=w386:bool, "VCluster out"=w395:variant)  [unwired: 5 in]
              n132 = Variant To Data(error in=w396, type=w391, Variant=w395) -> (data=w392:T1, error out=w387:errorcluster)
              n133 = Bundle By Name(cluster=w394, "VelocityFFG"=w392) -> (w393:refnum<class "Tapedrive_ESP301.lvclass">)
            }
            frame "AccelerationFFG" {
              n134 = call <instrlib>:"Set Acceleration Feed-Forward Gain.vi"("error in (no error)"=w423, "Acceleration feed-forward gain factor (0)"=w422, "Axis (1)"=w420, "VISA resource name"=w426) -> ("error out"=w421:errorcluster, "VISA resource name out"=w425:refnum<visa-resource-name>)  [unwired: 2 in]
              n135 = Unbundle By Name(w413) -> ("AccelerationFFG"=w419:T1)
              n136 = call "Get Acceleration Feed-Forward Gain_CK.vi"("error in (no error)"=w421, "Wait before read (0ms)"=w406, "Axis (1)"=w420, "VISA resource name"=w425) -> ("error out"=w409:errorcluster, "Gain"=w411:dbl, "VISA resource name out"=w424:refnum<visa-resource-name>)  [unwired: 1 in]
              n137 = Concatenate Strings(w410, ".Value" ("string")) -> (w417:string)
              n138 = call "Set Cluster Element by Name__ogtk_TS.vi"("error in (no error)"=w409, "Element Name (\"\": New Element Data Name)"=w417, "New Element Value"=w411, "Cluster"=w419) -> ("error out"=w416:errorcluster, "found?"=w407:bool, "VCluster out"=w415:variant)  [unwired: 5 in]
              n139 = Variant To Data(error in=w416, type=w419, Variant=w415) -> (data=w414:T1, error out=w408:errorcluster)
              n140 = Bundle By Name(cluster=w413, "AccelerationFFG"=w414) -> (w412:refnum<class "Tapedrive_ESP301.lvclass">)
            }
          }
          "found?" <- w257
          n141 = call "createCommandListForCommandCase.vi"("immediate Check (only once)"=TRUE, "setvalue"=w273, "command"=w269) -> ("new commands"=w264:string)  [unwired: 8 in]
          n142 = call-poly "CompressAndUpdate_Poly.vi"("force CVT update (false)"=TRUE, "error in"=w267, "Numeric"=w268, "command or variable name"=w269) -> ("error out"=w259:errorcluster)  [unwired: 7 in]
          n143 = Bundle By Name(cluster=w262, "Connection"=w263) -> (w271:refnum<class "Tapedrive_ESP301.lvclass">)
        }
        frame "setDACoffset" {
          n144 = call "reBuildJoindCommand.vi"("number of group elements (0)"=1, "Args"=w464, "Command 2"=w456) -> ("Arg"=w460:string, "Command"=w427:string)
          n145 = Unbundle By Name(w458) -> ("Settings"=w442:T6, "forwardaxis"=w455:i16, "backwardaxis"=w454:i16)
          n146 = call "getSeperator.vi"("Channel Seperator (\"\")"=w462, "Command"=w427) -> ("Channel"=w439:string)  [unwired: 8 in, 1 out]
          n147 = call "CheckIfSetCommand.vi"("Command"=w427) -> ("variable"=w434:string)  [unwired: 2 out]
          n148 = Decimal String To Number(string=w439) -> (number=w453:i32)  [unwired: 2 in, 1 out]
          n149 = Build Array(w455, w454) -> (w451:i16[])
          n150 = Decrement(x=w453) -> (x-1=w452:i32)
          n151 = Fract/Exp String To Number(string=w460) -> (number=w461:dbl)  [unwired: 3 in, 1 out]
          n152 = Index Array(array=w451, index=w452) -> (element=w450:i16)
          n153 = Decrement(x=w450) -> (x-1=w447:i16)
          n154 = Multiply(x=2, y=w447) -> (x*y=w448:i32)
          n155 = Add(x=1, y=w448) -> (x+y=w445:i32)
          n156 = call <instrlib>:"Set DAC Offset.vi"("error in (no error)"=w465, "DAC Offset (0)"=w461, "Axis (1)"=w445, "VISA resource name"=w466) -> ("error out"=w443:errorcluster, "VISA resource name out"=w444:refnum<visa-resource-name>)  [unwired: 2 in]
          n157 = call "createCommandListForCommandCase.vi"("immediate Check (only once)"=TRUE, "setvalue"=w460) -> ("new commands"=w441:string)  [unwired: 9 in]
          n158 = Concatenate Strings("\nsetPower.Axis ", w439) -> (w436:string)
          n159 = Concatenate Strings(w436, ">>off ") -> (w431:string)
          n160 = Concatenate Strings("\nget" ("string"), w434) -> (w429:string)
          n161 = Concatenate Strings(w436, ">>on ") -> (w430:string)
          n162 = Concatenate Strings(w431, "\n", w430, w429) -> (w428:string)
          n163 = Bundle By Name(cluster=w458, "Settings"=w442, "Connection"=w444) -> (w457:refnum<class "Tapedrive_ESP301.lvclass">)
          n164 = Concatenate Strings(w441, w428) -> (w440:string)
        }
        frame "setMoveAcceleration", "setMoveDecceleration", "setMoveVelocity", "setTensionAcceleration", "setTensionDecceleration", "setTensionVelocity" {
          n165 = call "reBuildJoindCommand.vi"("number of group elements (0)"=1, "Args"=w487, "Command 2"=w480) -> ("Arg"=w485:string, "Command"=w479:string)
          n166 = Unbundle By Name(w483) -> ("Settings"=w472:T6)
          n167 = call "createCommandListForCommandCase.vi"("immediate Check (only once)"=TRUE, "setvalue"=w485, "command"=w479) -> ("new commands"=w477:string)  [unwired: 8 in]
          n168 = call "CheckIfSetCommand.vi"("Command"=w479) -> ("variable"=w473:string)  [unwired: 2 out]
          n169 = Fract/Exp String To Number(string=w485) -> (number=w471:dbl)  [unwired: 3 in, 1 out]
          n170 = Concatenate Strings(w473, ".Value" ("string")) -> (w468:string)
          n171 = call-poly "CompressAndUpdate_Poly.vi"("force CVT update (false)"=TRUE, "error in"=w476, "Numeric"=w471, "command or variable name"=w479) -> ("error out"=w470:errorcluster)  [unwired: 7 in]
          n172 = call "Set Cluster Element by Name__ogtk_TS.vi"("error in (no error)"=w470, "Element Name (\"\": New Element Data Name)"=w468, "New Element Value"=w471, "Cluster"=w472) -> ("error out"=w467:errorcluster, "VCluster out"=w469:variant)  [unwired: 5 in, 1 out]
          n173 = Variant To Data(error in=w467, type=w472, Variant=w469) -> (data=w482:T6, error out=w475:errorcluster)
          n174 = Bundle By Name(cluster=w483, "Settings"=w482) -> (w481:refnum<class "Tapedrive_ESP301.lvclass">)
        }
        frame "getAcceleration", "getAccelerationFFG", "getDACoffset", "getDecceleration", "getMaxAcceleration", "getMaxVelocity", "getVelocity", "getVelocityFFG" {
          n175 = Unbundle By Name(w493) -> ("forwardaxis"=w499:i16, "backwardaxis"=w498:i16)
          n176 = call "reBuildJoindCommand.vi"("number of group elements (0)"=1, "Args"=w515, "Command 2"=w504) -> ("Arg"=w511:string, "Command"=w489:string)
          n177 = call "getSeperator.vi"("Channel Seperator (\"\")"=w513, "Command"=w489) -> ("Channel"=w512:string, "Seperator (e.g. \"Channel1\")"=w490:string)  [unwired: 8 in]
          n178 = Decimal String To Number(string=w512) -> (number=w497:i32)  [unwired: 2 in, 1 out]
          n179 = Decrement(x=w497) -> (x-1=w496:i32)
          n180 = Build Array(w499, w498) -> (w495:i16[])
          n181 = Index Array(array=w495, index=w496) -> (element=w494:i16)
          n182 = call "CheckIfSetCommand.vi"("Command"=w504) -> ("variable"=w503:string)  [unwired: 2 out]
          n183 = case shown="\"MaxVelocity\"" w503 {
            tunnel: w505 -> [w529 w544 w561 w578 w592 w608 w624 w642]
            tunnel: w506 -> [w528 w545 w560 w577 w594 w609 w625 w644]
            tunnel: w494 -> [w530 w547 w562 w576 w593 w610 w626 w645]
            tunnel: [w517 w532 w550 w564 w580 w598 w613 w632] -> w502
            tunnel: [w516 w534 w549 w567 w583 w596 w612 w633] -> w501
            tunnel: [w531 w546 w563 w579 w595 w611 w627 w643] -> w507
            tunnel: w493 -> [w521 w537 w552 w569 w585 w601 w617 w631]
            tunnel: [w520 w538 w553 w568 w584 w600 w616 w630] -> w492
            tunnel: w490 -> [w519 w535 w548 w566 w581 w602 w614 w629]
            frame "Velocity", Default {
              n184 = Unbundle By Name(w521) -> ("Velocity"=w526:T1)
              n185 = call "Get Velocity_CK.vi"("error in (no error)"=w528, "Axis (1)"=w530, "VISA resource name"=w529) -> ("error out"=w518:errorcluster, "Velocity (units/s)"=w516:dbl, "VISA resource name out"=w531:refnum<visa-resource-name>)  [unwired: 2 in]
              n186 = Concatenate Strings(w519, ".Value" ("string")) -> (w523:string)
              n187 = call "Set Cluster Element by Name__ogtk_TS.vi"("error in (no error)"=w518, "Element Name (\"\": New Element Data Name)"=w523, "New Element Value"=w516, "Cluster"=w526) -> ("error out"=w524:errorcluster, "VCluster out"=w525:variant)  [unwired: 5 in, 1 out]
              n188 = Variant To Data(error in=w524, type=w526, Variant=w525) -> (data=w527:T1, error out=w517:errorcluster)
              n189 = Bundle By Name(cluster=w521, "Velocity"=w527) -> (w520:refnum<class "Tapedrive_ESP301.lvclass">)
            }
            frame "Acceleration" {
              n190 = Unbundle By Name(w537) -> ("Acceleration"=w536:T1)
              n191 = call "Get Acceleration_CK.vi"("error in (no error)"=w545, "Axis (1)"=w547, "VISA resource name"=w544) -> ("error out"=w533:errorcluster, "Acceleration (units/s²)"=w534:dbl, "VISA resource name out"=w546:refnum<visa-resource-name>)  [unwired: 2 in]
              n192 = Concatenate Strings(w535, ".Value" ("string")) -> (w540:string)
              n193 = call "Set Cluster Element by Name__ogtk_TS.vi"("error in (no error)"=w533, "Element Name (\"\": New Element Data Name)"=w540, "New Element Value"=w534, "Cluster"=w536) -> ("error out"=w541:errorcluster, "VCluster out"=w542:variant)  [unwired: 5 in, 1 out]
              n194 = Variant To Data(error in=w541, type=w536, Variant=w542) -> (data=w543:T1, error out=w532:errorcluster)
              n195 = Bundle By Name(cluster=w537, "Acceleration"=w543) -> (w538:refnum<class "Tapedrive_ESP301.lvclass">)
            }
            frame "Decceleration" {
              n196 = Unbundle By Name(w552) -> ("Decceleration"=w558:T1)
              n197 = call "Get Deceleration_CK.vi"("error in (no error)"=w560, "Axis (1)"=w562, "VISA resource name"=w561) -> ("error out"=w551:errorcluster, "Deceleration (units/s²)"=w549:dbl, "VISA resource name out"=w563:refnum<visa-resource-name>)  [unwired: 2 in]
              n198 = Concatenate Strings(w548, ".Value" ("string")) -> (w555:string)
              n199 = call "Set Cluster Element by Name__ogtk_TS.vi"("error in (no error)"=w551, "Element Name (\"\": New Element Data Name)"=w555, "New Element Value"=w549, "Cluster"=w558) -> ("error out"=w556:errorcluster, "VCluster out"=w557:variant)  [unwired: 5 in, 1 out]
              n200 = Variant To Data(error in=w556, type=w558, Variant=w557) -> (data=w559:T1, error out=w550:errorcluster)
              n201 = Bundle By Name(cluster=w552, "Decceleration"=w559) -> (w553:refnum<class "Tapedrive_ESP301.lvclass">)
            }
            frame "MaxVelocity" {
              n202 = Unbundle By Name(w569) -> ("MaxVelocity"=w574:T1)
              n203 = call "Get Maximum Velocity_CK.vi"("error in (no error)"=w577, "Axis (1)"=w576, "VISA resource name"=w578) -> ("error out"=w565:errorcluster, "Maximum Velocity (units/s)"=w567:dbl, "VISA resource name out"=w579:refnum<visa-resource-name>)  [unwired: 2 in]
              n204 = Concatenate Strings(w566, ".Value" ("string")) -> (w571:string)
              n205 = call "Set Cluster Element by Name__ogtk_TS.vi"("error in (no error)"=w565, "Element Name (\"\": New Element Data Name)"=w571, "New Element Value"=w567, "Cluster"=w574) -> ("error out"=w572:errorcluster, "VCluster out"=w573:variant)  [unwired: 5 in, 1 out]
              n206 = Variant To Data(error in=w572, type=w574, Variant=w573) -> (data=w575:T1, error out=w564:errorcluster)
              n207 = Bundle By Name(cluster=w569, "MaxVelocity"=w575) -> (w568:refnum<class "Tapedrive_ESP301.lvclass">)
            }
            frame "MaxAcceleration" {
              n208 = Unbundle By Name(w585) -> ("MaxAcceleration"=w590:T1)
              n209 = call "Get Maximum Acceleration and Deceleration_CK.vi"("error in (no error)"=w594, "Axis (1)"=w593, "VISA resource name"=w592) -> ("error out"=w582:errorcluster, "Acceleration (units/s²)"=w583:dbl, "VISA resource name out"=w595:refnum<visa-resource-name>)  [unwired: 2 in]
              n210 = Concatenate Strings(w581, ".Value" ("string")) -> (w587:string)
              n211 = call "Set Cluster Element by Name__ogtk_TS.vi"("error in (no error)"=w582, "Element Name (\"\": New Element Data Name)"=w587, "New Element Value"=w583, "Cluster"=w590) -> ("error out"=w588:errorcluster, "VCluster out"=w589:variant)  [unwired: 5 in, 1 out]
              n212 = Variant To Data(error in=w588, type=w590, Variant=w589) -> (data=w591:T1, error out=w580:errorcluster)
              n213 = Bundle By Name(cluster=w585, "MaxAcceleration"=w591) -> (w584:refnum<class "Tapedrive_ESP301.lvclass">)
            }
            frame "VelocityFFG" {
              n214 = Unbundle By Name(w601) -> ("VelocityFFG"=w597:T1)
              n215 = call "Get Velocity Feed-Forward Gain_CK.vi"("error in (no error)"=w609, "Axis (1)"=w610, "VISA resource name"=w608) -> ("error out"=w599:errorcluster, "Gain"=w596:dbl, "VISA resource name out"=w611:refnum<visa-resource-name>)  [unwired: 2 in]
              n216 = Concatenate Strings(w602, ".Value" ("string")) -> (w604:string)
              n217 = call "Set Cluster Element by Name__ogtk_TS.vi"("error in (no error)"=w599, "Element Name (\"\": New Element Data Name)"=w604, "New Element Value"=w596, "Cluster"=w597) -> ("error out"=w605:errorcluster, "VCluster out"=w606:variant)  [unwired: 5 in, 1 out]
              n218 = Variant To Data(error in=w605, type=w597, Variant=w606) -> (data=w607:T1, error out=w598:errorcluster)
              n219 = Bundle By Name(cluster=w601, "VelocityFFG"=w607) -> (w600:refnum<class "Tapedrive_ESP301.lvclass">)
            }
            frame "AccelerationFFG" {
              n220 = Unbundle By Name(w617) -> ("AccelerationFFG"=w622:T1)
              n221 = call "Get Acceleration Feed-Forward Gain_CK.vi"("error in (no error)"=w625, "Axis (1)"=w626, "VISA resource name"=w624) -> ("error out"=w615:errorcluster, "Gain"=w612:dbl, "VISA resource name out"=w627:refnum<visa-resource-name>)  [unwired: 2 in]
              n222 = Concatenate Strings(w614, ".Value" ("string")) -> (w619:string)
              n223 = call "Set Cluster Element by Name__ogtk_TS.vi"("error in (no error)"=w615, "Element Name (\"\": New Element Data Name)"=w619, "New Element Value"=w612, "Cluster"=w622) -> ("error out"=w620:errorcluster, "VCluster out"=w621:variant)  [unwired: 5 in, 1 out]
              n224 = Variant To Data(error in=w620, type=w622, Variant=w621) -> (data=w623:T1, error out=w613:errorcluster)
              n225 = Bundle By Name(cluster=w617, "AccelerationFFG"=w623) -> (w616:refnum<class "Tapedrive_ESP301.lvclass">)
            }
            frame "DACoffset" {
              n226 = Unbundle By Name(w631) -> ("DACoffset"=w639:T1)
              n227 = Decrement(x=w645) -> (x-1=w647:i16)
              n228 = Multiply(x=2, y=w647) -> (x*y=w648:i32)
              n229 = Add(x=1, y=w648) -> (x+y=w641:i32)
              n230 = call "Get DAC Offset_CK.vi"("error in (no error)"=w644, "Wait before read (0ms)"=u32 100, "Axis (1)"=w641, "VISA resource name"=w642) -> ("error out"=w634:errorcluster, "DAC Offset"=w633:dbl, "VISA resource name out"=w643:refnum<visa-resource-name>)  [unwired: 1 in]
              n231 = Concatenate Strings(w629, ".Value" ("string")) -> (w636:string)
              n232 = call "Set Cluster Element by Name__ogtk_TS.vi"("error in (no error)"=w634, "Element Name (\"\": New Element Data Name)"=w636, "New Element Value"=w633, "Cluster"=w639) -> ("error out"=w637:errorcluster, "VCluster out"=w638:variant)  [unwired: 5 in, 1 out]
              n233 = Variant To Data(error in=w637, type=w639, Variant=w638) -> (data=w640:T1, error out=w632:errorcluster)
              n234 = Bundle By Name(cluster=w631, "DACoffset"=w640) -> (w630:refnum<class "Tapedrive_ESP301.lvclass">)
            }
          }
          n235 = call "createCommandListForCommandCase.vi"("immediate Check (only once)"=TRUE, "setvalue"=w511, "command"=w489) -> ("new commands"=w509:string)  [unwired: 8 in]
          n236 = Bundle By Name(cluster=w492, "Connection"=w507) -> (w508:refnum<class "Tapedrive_ESP301.lvclass">)
          n237 = call "CheckIfSetCommand.vi"("Command"=w489) -> ("variable"=w488:string)  [unwired: 2 out]
          n238 = call-poly "CompressAndUpdate_Poly.vi"("force CVT update (false)"=TRUE, "error in"=w502, "Numeric"=w501, "command or variable name"=w488) -> ("error out"=w491:errorcluster)  [unwired: 7 in]
        }
        frame "setPower" {
          n239 = call "reBuildJoindCommand.vi"("number of group elements (0)"=1, "Args"=w673, "Command 2"=w687) -> ("Arg"=w683:string, "Command"=w664:string)
          n240 = Unbundle By Name(w680) -> ("Settings"=w658:T6, "forwardaxis"=w655:i16, "backwardaxis"=w654:i16)
          n241 = call "getSeperator.vi"("Channel Seperator (\"\")"=w685, "Command"=w664) -> ("Channel"=w684:string)  [unwired: 8 in, 1 out]
          n242 = Decimal String To Number(string=w684) -> (number=w651:i32)  [unwired: 2 in, 1 out]
          n243 = Index Array(array=w673, index=0) -> (element=w674:string)
          n244 = Decrement(x=w651) -> (x-1=w650:i32)
          n245 = case shown="\"on\"" w674 {
            tunnel: [FALSE TRUE] -> w666
            frame "off", Default {
            }
            frame "on" {
            }
          }
          n246 = Build Array(w655, w654) -> (w652:i16[])
          n247 = Index Array(array=w652, index=w650) -> (element=w653:i16)
          n248 = call <instrlib>:"Enable Disable Motor.vi"("error in (no error)"=w676, "Action (OFF)"=w666, "Axis (1)"=w653, "VISA resource name"=w677) -> ("error out"=w671:errorcluster, "VISA resource name out"=w672:refnum<visa-resource-name>)  [unwired: 2 in]
          n249 = call "Get Motor Power Status_CK.vi"("error in (no error)"=w671, "Axis (1)"=w653, "VISA resource name"=w672) -> ("error out"=w665:errorcluster, "Power Status"=w667:bool, "VISA resource name out"=w670:refnum<visa-resource-name>)  [unwired: 2 in]
          n250 = call "createCommandListForCommandCase.vi"("immediate Check (only once)"=TRUE, "setvalue"=w683, "command"=w664) -> ("new commands"=w681:string)  [unwired: 8 in]
          n251 = Select(t=OnOffTypeDef."on" ("Settings.inmotion"), s=w667, f=OnOffTypeDef."off" ("Settings.inmotion")) -> (s? t:f=w656:T3)
          n252 = call "CheckIfSetCommand.vi"("Command"=w664) -> ("variable"=w657:string)  [unwired: 2 out]
          n253 = call-poly "CompressAndUpdate_Poly.vi"("force CVT update (false)"=TRUE, "error in"=w665, "enum variant"=w656, "command or variable name"=w664) -> ("error out"=w661:errorcluster)  [unwired: 7 in]
          n254 = call "Set Cluster Element by Name__ogtk_TS.vi"("error in (no error)"=w661, "Element Name (\"\": New Element Data Name)"=w657, "New Element Value"=w656, "Cluster"=w658) -> ("error out"=w660:errorcluster, "VCluster out"=w659:variant)  [unwired: 5 in, 1 out]
          n255 = Variant To Data(error in=w660, type=w658, Variant=w659) -> (data=w679:T6, error out=w662:errorcluster)
          n256 = Bundle By Name(cluster=w680, "Settings"=w679, "Connection"=w670) -> (w678:refnum<class "Tapedrive_ESP301.lvclass">)
        }
        frame "getPower" {
          n257 = call "reBuildJoindCommand.vi"("number of group elements (0)"=1, "Args"=w708, "Command 2"=w717) -> ("Arg"=w713:string, "Command"=w690:string)
          n258 = call "getSeperator.vi"("Channel Seperator (\"\")"=w715, "Command"=w690) -> ("Channel"=w714:string, "Seperator (e.g. \"Channel1\")"=w691:string)  [unwired: 8 in]
          n259 = Decimal String To Number(string=w714) -> (number=w707:i32)  [unwired: 2 in, 1 out]
          n260 = call "Get Motor Power Status_CK.vi"("error in (no error)"=w701, "Axis (1)"=w707, "VISA resource name"=w702) -> ("error out"=w700:errorcluster, "Power Status"=w703:bool, "VISA resource name out"=w706:refnum<visa-resource-name>)  [unwired: 2 in]
          n261 = Unbundle By Name(w693) -> ("Power"=w692:cluster{"Axis 1":T3, "Axis 2":T3})
          n262 = Select(t=OnOffTypeDef."on" ("Settings.inmotion"), s=w703, f=OnOffTypeDef."off" ("Settings.inmotion")) -> (s? t:f=w694:T3)
          n263 = call "createCommandListForCommandCase.vi"("immediate Check (only once)"=TRUE, "setvalue"=w713, "command"=w690) -> ("new commands"=w711:string)  [unwired: 8 in]
          n264 = call-poly "CompressAndUpdate_Poly.vi"("force CVT update (false)"=TRUE, "error in"=w700, "enum variant"=w694, "command or variable name"=w690) -> ("error out"=w696:errorcluster)  [unwired: 7 in]
          n265 = call "Set Cluster Element by Name__ogtk_TS.vi"("error in (no error)"=w696, "Element Name (\"\": New Element Data Name)"=w691, "New Element Value"=w694, "Cluster"=w692) -> ("error out"=w697:errorcluster, "VCluster out"=w695:variant)  [unwired: 5 in, 1 out]
          n266 = Variant To Data(error in=w697, type=w692, Variant=w695) -> (data=w710:cluster{"Axis 1":T3, "Axis 2":T3}, error out=w698:errorcluster)
          n267 = Bundle By Name(cluster=w693, "Power"=w710, "Connection"=w706) -> (w709:refnum<class "Tapedrive_ESP301.lvclass">)
        }
        frame "putMasterSlave" {
          n268 = Index Array(array=w723) -> (element=w722:string)  [unwired: 1 in]
          n269 = call "MASTERSLAVE.vi"("error in (no error)"=w721, "Arg"=w722, "Tapedrive_ESP301 in"=w720) -> ("error out"=w718:errorcluster, "Tapedrive_ESP301 out"=w719:refnum<class "Tapedrive_ESP301.lvclass">)  [unwired: 7 in]
        }
        frame "putReleaseSlaving" {
          n270 = call "releaseSlaving.vi"("error in (no error)"=w727, "Tapedrive_ESP301 in"=w726) -> ("error out"=w724:errorcluster, "Tapedrive_ESP301 out"=w725:refnum<class "Tapedrive_ESP301.lvclass">)  [unwired: 8 in]
        }
        frame "Wait" {
          n271 = Index Array(array=w731) -> (element=w730:string)  [unwired: 1 in]
          n272 = Fract/Exp String To Number(string=w730) -> (number=w729:dbl)  [unwired: 3 in, 1 out]
          n273 = To Unsigned Long Integer(number=w729) -> (unsigned 32bit integer=w728:u32)
          n274 = Wait (ms)(milliseconds to wait=w728) -> ()  [unwired: 1 out]
        }
        frame "putStep" {
          n275 = call "checkSettingsClass.vi"("Tapedrive_ESP301 in"=w737) -> ("forwardaxis"=w735:i16, "settings needed"=w745:bool, "spreadsheet string"=w744:string, "Tension"=w738:T3)  [unwired: 6 in, 1 out]
          n276 = case shown="\"on\"" w738 {
            tunnel: w742 -> [w747 w750]
            tunnel: [w747 w749] -> w741
            tunnel: w740 -> [w746 w753]
            tunnel: w735 -> [_ w752]
            tunnel: [w746 w748] -> w739
            frame "off", Default {
            }
            frame "on" {
              n277 = call <instrlib>:"Stop Motion.vi"("error in (no error)"=w750, "Stop all axes (F)"=TRUE, "Axis (1)"=w752, "VISA resource name"=w753) -> ("error out"=w749:errorcluster, "VISA resource name out"=w748:refnum<visa-resource-name>)  [unwired: 2 in]
            }
          }
          n278 = case shown="False" w745 {
            tunnel: w744 -> [_ w794]
            tunnel: [w758 w793] -> w743
            tunnel: w741 -> [w778 w795]
            tunnel: w739 -> [w777 w790]
            tunnel: w737 -> [w781 w792]
            tunnel: [w761 w791] -> w734
            tunnel: [w759 w795] -> w736
            frame False {
              # "todo updater CVT?Cluster - rewrite log"
              n279 = Unbundle By Name(w781) -> ("targetpos"=w755:dbl, "Value"=w754:dbl, "Value"=w780:dbl, "forwardaxis"=w757:i16, "backwardaxis"=w779:i16, "Direction"=w765:T5)
              n280 = call "direction_axis.vi"("Direction"=w765, "backwardaxis"=w779, "forwardaxis"=w757) -> ("Slave"=w767:i16, "Master"=w756:i16)  [unwired: 7 in]
              n281 = call <instrlib>:"Set Master-Slave Reduction Ratio.vi"("error in (no error)"=w778, "Reduction Ratio (0)"=0.0, "Axis (1)"=w767, "VISA resource name"=w777) -> ("error out"=w775:errorcluster, "VISA resource name out"=w774:refnum<visa-resource-name>)  [unwired: 2 in]
              n282 = call <instrlib>:"Get Master-Slave Reduction Ratio.vi"("error in (no error)"=w775, "Axis (1)"=w767, "VISA resource name"=w774) -> ("error out"=w771:errorcluster, "Reduction Ratio"=w768:dbl, "VISA resource name out"=w773:refnum<visa-resource-name>)  [unwired: 2 in]
              n283 = call-poly "CompressAndUpdate_Poly.vi"("force CVT update (false)"=TRUE, "error in"=w771, "Numeric"=w768, "command or variable name"="RedRatio") -> ("error out"=w770:errorcluster)  [unwired: 7 in]
              n284 = Equal?(x=w757, y=w756) -> ()  [unwired: 1 out]
              n285 = flat-sequence {
                tunnel: w754 -> [w788]
                tunnel: [w787] -> w760
                tunnel: w773 -> [w786]
                tunnel: w770 -> [w785]
                tunnel: [w784] -> w766
                tunnel: [w783] -> w763
                tunnel: w756 -> [w782]
                frame #0 {
                  n286 = Tick Count (ms)() -> (millisecond timer value=w784:u32)
                  n287 = call <instrlib>:"Move Relative.vi"("error in (no error)"=w785, "Position (0 units)"=w788, "Axis (1)"=w782, "VISA resource name"=w786) -> ("error out"=w787:errorcluster, "VISA resource name out"=w783:refnum<visa-resource-name>)  [unwired: 2 in]
                }
              }
              n288 = Bundle By Name(cluster=w781, "targetpos"=w755, "startpos"=w780, "startTime"=w766, "Moving?"=TRUE ("Wait for Step"), "Connection"=w763) -> (w762:refnum<class "Tapedrive_ESP301.lvclass">)
              n289 = call-dynamic "QuickCheckStop.vi"("error in (no error)"=w760, "Tapedrive Object"=w762) -> ("error out (no error)"=w759:errorcluster, "new commands"=w758:string, "Tapedrive Object 2"=w761:refnum<class "Tapedrive_ESP301.lvclass">)  [unwired: 7 in]
            }
            frame True {
              n290 = disable-structure shown="Enabled" {
                disable-tunnel: w794 -> [w799 w800]
                disable-tunnel: [w796 w800] -> w793
                frame Enabled {
                  n291 = Concatenate Strings(w799, "\n", "putStep") -> (w796:string)
                }
                frame Disabled {
                }
              }
              n292 = Bundle By Name(cluster=w792, "Connection"=w790, "Moving?"=FALSE) -> (w791:refnum<class "Tapedrive_ESP301.lvclass">)
            }
          }
        }
        frame "setReductionRatio" {
          n293 = Unbundle By Name(w811) -> ("forwardaxis"=w818:i16, "backwardaxis"=w817:i16, "Direction"=w816:T5)
          n294 = Index Array(array=w814) -> (element=w813:string)  [unwired: 1 in]
          n295 = Fract/Exp String To Number(string=w813) -> (number=w812:dbl)  [unwired: 3 in, 1 out]
          n296 = call "direction_axis.vi"("Direction"=w816, "backwardaxis"=w817, "forwardaxis"=w818) -> ("Slave"=w807:i16)  [unwired: 7 in, 1 out]
          n297 = call <instrlib>:"Set Master-Slave Reduction Ratio.vi"("error in (no error)"=w815, "Reduction Ratio (0)"=w812, "Axis (1)"=w807, "VISA resource name"=w819) -> ("error out"=w808:errorcluster, "VISA resource name out"=w809:refnum<visa-resource-name>)  [unwired: 2 in]
          n298 = call <instrlib>:"Get Master-Slave Reduction Ratio.vi"("error in (no error)"=w808, "Axis (1)"=w807, "VISA resource name"=w809) -> ("error out"=w805:errorcluster, "Reduction Ratio"=w801:dbl, "VISA resource name out"=w806:refnum<visa-resource-name>)  [unwired: 2 in]
          n299 = call-poly "CompressAndUpdate_Poly.vi"("force CVT update (false)"=TRUE, "error in"=w805, "Numeric"=w801, "command or variable name"=w803) -> ("error out"=w804:errorcluster)  [unwired: 7 in]
          n300 = Bundle By Name(cluster=w811, "Connection"=w806, "Value"=w801) -> (w810:refnum<class "Tapedrive_ESP301.lvclass">)
        }
        frame "putTension" {
          n301 = Unbundle By Name(w825) -> ("Velocity"=w841:T1, "Acceleration"=w840:T1, "Decceleration"=w839:T1, "TensionVelocity"=w838:T1, "TensionAcceleration"=w837:T1, "TensionDecceleration"=w836:T1, "Tension"=w826:T3, "forwardaxis"=w820:i16)
          n302 = Build Array(w841, w840, w839) -> (w835:T7)
          n303 = Build Array(w838, w837, w836) -> (w834:T7)
          n304 = case shown="\"on\"" w826 {
            tunnel: w830 -> [w844 w847]
            tunnel: [w844 w846] -> w829
            tunnel: w828 -> [w843 w850]
            tunnel: w820 -> [_ w849]
            tunnel: [w843 w845] -> w827
            frame "off", Default {
            }
            frame "on" {
              n305 = call <instrlib>:"Stop Motion.vi"("error in (no error)"=w847, "Stop all axes (F)"=TRUE, "Axis (1)"=w849, "VISA resource name"=w850) -> ("error out"=w846:errorcluster, "VISA resource name out"=w845:refnum<visa-resource-name>)  [unwired: 2 in]
            }
          }
          n306 = call "set_Mode.vi"("Array"=w834, "Array 3"=string[] ["Velocity", "Acceleration", "Decceleration"], "Array 2"=w835) -> ("settings needed"=w833:bool, "spreadsheet string"=w832:string)  [unwired: 7 in]
          n307 = case shown="False" w833 {
            tunnel: w832 -> [_ w878]
            tunnel: ["" w881] -> w831
            tunnel: w829 -> [w865 w883]
            tunnel: w827 -> [w864 w882]
            tunnel: w825 -> [w875 w884]
            tunnel: [w874 w884] -> w823
            tunnel: [w852 w883] -> w824
            tunnel: [w870 w882] -> w821
            frame False {
              n308 = Unbundle By Name(w875) -> ("Value"=w872:dbl, "Value"=w873:dbl, "forwardaxis"=w866:i16, "backwardaxis"=w867:i16, "Direction"=w871:T5, "Value"=w851:dbl)
              n309 = call "direction_axis.vi"("Direction"=w871, "backwardaxis"=w867, "forwardaxis"=w866) -> ("Slave"=w854:i16, "Master"=w868:i16)  [unwired: 7 in]
              n310 = call <instrlib>:"Set Master-Slave Reduction Ratio.vi"("error in (no error)"=w865, "Reduction Ratio (0)"=1.0, "Axis (1)"=w854, "VISA resource name"=w864) -> ("error out"=w860:errorcluster, "VISA resource name out"=w862:refnum<visa-resource-name>)  [unwired: 2 in]
              n311 = call <instrlib>:"Get Master-Slave Reduction Ratio.vi"("error in (no error)"=w860, "Axis (1)"=w854, "VISA resource name"=w862) -> ("error out"=w859:errorcluster, "Reduction Ratio"=w857:dbl, "VISA resource name out"=w861:refnum<visa-resource-name>)  [unwired: 2 in]
              n312 = call-poly "CompressAndUpdate_Poly.vi"("force CVT update (false)"=TRUE, "error in"=w859, "Numeric"=w857, "command or variable name"="RedRatio") -> ("error out"=w858:errorcluster)  [unwired: 7 in]
              n313 = Bundle By Name(cluster=w875, "startpos"=w873) -> (w874:refnum<class "Tapedrive_ESP301.lvclass">)
              n314 = call <instrlib>:"Move Relative.vi"("error in (no error)"=w858, "Position (0 units)"=w872, "Axis (1)"=w868, "VISA resource name"=w861) -> ("error out"=w853:errorcluster, "VISA resource name out"=w870:refnum<visa-resource-name>)  [unwired: 2 in]
              n315 = flat-sequence {
                tunnel: w853 -> [w877]
                tunnel: [w877] -> w852
                tunnel: w851 -> [w876]
                frame #0 {
                  n316 = Wait (ms)(milliseconds to wait=w876) -> ()  [unwired: 1 out]
                }
              }
            }
            frame True {
              n317 = Concatenate Strings(w878, "\n", "putTension") -> (w881:string)
              "spreadsheet string" <- w878
            }
          }
          n318 = Bundle By Name(cluster=w823, "Connection"=w821) -> (w822:refnum<class "Tapedrive_ESP301.lvclass">)
        }
        frame "setDirection" {
          n319 = Unbundle By Name(w897) -> ("forwardaxis"=w903:i16, "Tension"=w901:T3)  [unwired: 1 out]
          n320 = Index Array(array=w905) -> (element=w896:string)  [unwired: 1 in]
          n321 = case shown="\"Moving\"" T4."Moving" ("status") {
            tunnel: w904 -> [w916 w924]
            tunnel: w903 -> [_ w923]
            tunnel: w902 -> [w915 w921]
            tunnel: [w915 w918] -> w898
            tunnel: [w916 w920] -> _
            frame Default {
            }
            frame "Moving" {
              n322 = call <instrlib>:"Stop Motion.vi"("error in (no error)"=w921, "Stop all axes (F)"=TRUE, "Axis (1)"=w923, "VISA resource name"=w924) -> ("error out"=w919:errorcluster, "VISA resource name out"=w920:refnum<visa-resource-name>)  [unwired: 2 in]
              n323 = call <userlib>:"Wait (ms)__ogtk.vi"("error in (no error)"=w919, "milliseconds to wait"=u32 300) -> ("error out"=w918:errorcluster)  [unwired: 8 in, 1 out]
            }
          }
          n324 = disable-structure shown="Disabled" {
            disable-tunnel: w901 -> [w909 _]
            disable-tunnel: [w907 _] -> w900
            disable-tunnel: w896 -> [w906 _]
            frame Disabled {
              n325 = Concatenate Strings("putReleaseSlaving\nputMasterSlave>>", w906) -> (w908:string)
              n326 = case shown="\"on\"" w909 {
                tunnel: w908 -> [w911 w914]
                tunnel: [w911 w912] -> w907
                frame "off", Default {
                }
                frame "on" {
                  n327 = Concatenate Strings(w914, "putTension" ("string")) -> (w912:string)
                }
              }
            }
            frame Enabled {
            }
          }
          n328 = disable-structure shown="Disabled" {
            frame Disabled {
            }
            frame Enabled {
            }
          }
          n329 = call "releaseSlaving.vi"("error in (no error)"=w898, "Tapedrive_ESP301 in"=w897) -> ("error out"=w895:errorcluster, "Tapedrive_ESP301 out"=w894:refnum<class "Tapedrive_ESP301.lvclass">)  [unwired: 8 in]
          n330 = call "MASTERSLAVE.vi"("error in (no error)"=w895, "Arg"=w896, "Tapedrive_ESP301 in"=w894) -> ("error out"=w891:errorcluster, "Tapedrive_ESP301 out"=w893:refnum<class "Tapedrive_ESP301.lvclass">)  [unwired: 7 in]
          n331 = call "SetTension.vi"("command"=enum16{"Move", "Tension"}."Tension", "error in (no error)"=w891, "Tapedrive_ESP301 in"=w893) -> ("error out"=w890:errorcluster, "Tapedrive_ESP301 out"=w888:refnum<class "Tapedrive_ESP301.lvclass">)  [unwired: 7 in]
          n332 = Unbundle By Name(w888) -> ("Connection"=w887:refnum<visa-resource-name>)
          n333 = call <instrlib>:"Error Query.vi"("error in (no error)"=w890, "VISA resource name"=w887) -> ("error out"=w889:errorcluster, "Error Message"=→"Error Message":string, "Error Code"=→"Error Code":i32[])  [unwired: 3 out]
        }
        frame "Abort" {
          n334 = Index Array(array=w926) -> (element=w925:string)  [unwired: 1 in]
          n335 = case shown="Default" w925 {
            tunnel: [w932 w955] -> w931
            tunnel: w930 -> [w932 w954]
            tunnel: w929 -> [_ w953]
            tunnel: w928 -> [w933 w952]
            tunnel: [w933 w938] -> w927
            frame "ClearQueue" {
            }
            frame Default {
              w937 = TRUE ("force CVT update (false)")
              w941 = FALSE ("Action (OFF)")
              n336 = Unbundle By Name(w954) -> ("forwardaxis"=w946:i16, "backwardaxis"=w945:i16)
              n337 = call <instrlib>:"Stop Motion.vi"("error in (no error)"=w952, "Stop all axes (F)"=TRUE, "Axis (1)"=w946, "VISA resource name"=w953) -> ("error out"=w949:errorcluster, "VISA resource name out"=w950:refnum<visa-resource-name>)  [unwired: 2 in]
              n338 = call <instrlib>:"Enable Disable Motor.vi"("error in (no error)"=w949, "Action (OFF)"=w941, "Axis (1)"=w946, "VISA resource name"=w950) -> ("error out"=w948:errorcluster, "VISA resource name out"=w944:refnum<visa-resource-name>)  [unwired: 2 in]
              n339 = call <instrlib>:"Enable Disable Motor.vi"("error in (no error)"=w948, "Action (OFF)"=w941, "Axis (1)"=w945, "VISA resource name"=w944) -> ("error out"=w940:errorcluster, "VISA resource name out"=w947:refnum<visa-resource-name>)  [unwired: 2 in]
              n340 = Bundle By Name(cluster=w954, "Connection"=w947) -> (w955:refnum<class "Tapedrive_ESP301.lvclass">)
              n341 = Select(t=OnOffTypeDef."on" ("Settings.inmotion"), s=w941, f=OnOffTypeDef."off" ("Settings.inmotion")) -> (s? t:f=w936:T3)
              n342 = call-poly "CompressAndUpdate_Poly.vi"("force CVT update (false)"=w937, "error in"=w940, "enum variant"=w936, "command or variable name"="setPower.Axis 1" ("Seperator out")) -> ("error out"=w939:errorcluster)  [unwired: 7 in]
              n343 = call-poly "CompressAndUpdate_Poly.vi"("force CVT update (false)"=w937, "error in"=w939, "enum variant"=w936, "command or variable name"="setPower.Axis 2" ("Seperator out")) -> ("error out"=w938:errorcluster)  [unwired: 7 in]
            }
          }
        }
      }
      n344 = case shown="True" w21 {
        tunnel: w25 -> [w27 w36]
        tunnel: [w27 w35] -> w24
        tunnel: [w28 w34] -> w18
        tunnel: w23 -> [w26 w33]
        tunnel: [w26 w32] -> w22
        tunnel: w9 -> [w29 w31]
        tunnel: [w29 w30] -> w20
        tunnel: w19 -> [w28 _]
        frame False {
        }
        frame True {
          n345 = call-parent "Configure.vi"("error in (no error)"=w33, "Msg in"=w31, "BaseDriver in"=w36) -> ("error out"=w32:errorcluster, "new command"=w34:string, "Msg out"=w30:T2, "BaseDriver out"=w35:refnum<class "Tapedrive_ESP301.lvclass">)  [unwired: 5 in]
        }
      }
    }
    frame Error {
    }
  }
  "error out" <- w5
  "FakePressureController out" <- w2
  "new command" <- w3
  "Msg out" <- w4
  n346 = disable-structure shown="Disabled" {
    frame Disabled {
      (unwired) OnOffTypeDef."off" ("inmotion")
      n347 = call <instrlib>:"Set Deceleration.vi"() -> ()  [unwired: 6 in, 2 out]
      n348 = call <instrlib>:"Set Velocity.vi"() -> ()  [unwired: 6 in, 2 out]
      n349 = call "CheckIfSetCommand.vi"() -> ()  [unwired: 1 in, 3 out]
      n350 = call <instrlib>:"Set Maximum Acceleration and Deceleration.vi"() -> ()  [unwired: 6 in, 2 out]
      n351 = call <instrlib>:"Set Maximum Velocity.vi"() -> ()  [unwired: 6 in, 2 out]
      n352 = call <instrlib>:"Get Master-Slave Velocity Update Interval.vi"() -> ()  [unwired: 5 in, 3 out]
      n353 = call "CheckIfSetCommand.vi"() -> ()  [unwired: 1 in, 3 out]
      n354 = call <instrlib>:"Get Master-Slave Velocity Update Interval.vi"() -> ()  [unwired: 5 in, 3 out]
    }
    frame Enabled {
    }
  }
  n355 = disable-structure shown="Disabled" {
    frame Disabled {
      n356 = call "GETVelocity.vi"() -> ()  [unwired: 10 in, 2 out]
      n357 = call "GETAcc.vi"() -> ()  [unwired: 10 in, 2 out]
      n358 = call "GETDAcc.vi"() -> ()  [unwired: 10 in, 2 out]
    }
    frame Enabled {
    }
  }
  n359 = Unbundle By Name(w2) -> ("Velocity"=→"Settings.Velocity":T1)
